vi "r3_Pick&Place_module_chip_Zoffset.vi"() -> ()   [LabVIEW 2016]
uses:
  Classes/Controllers/I-O/Copy of NI-DAQ Folder/NI-DAQ.lvclass
  D:/INTT/V1/Classes/Controllers/I-O/Copy of I-O Folder/I-O.lvclass
  Classes/Controllers/Dispenser/Copy of Ultimus V2 Folder/Ultimus V2.lvclass
  <vilib>/Analysis/coordinate.llb/2D Cartesian Coordinate Rotation (Scalar).vi
  <vilib>/Utility/file.llb/Read Delimited Spreadsheet (DBL).vi
  <vilib>/Utility/file.llb/Write Delimited Spreadsheet (DBL).vi
  Classes/Controllers/Motion/Copy of Motion Folder/Motion.lvclass
  Classes/Controllers/Camera/Copy of Controller Folder/Controller.lvclass
  <vilib>/Analysis/NI_AALPro.lvlib
  Classes/Controllers/I-O/Copy of I-O Folder/I-O.lvclass
panel:
  out "chip place Z offset":dbl[](array[numeric])
  out "air pressure indecator":i32
  in  "glue deposit group":i32=4
  in  "Ultimus Pressure":i16=20
  out "Array 2":dbl[][](array[numeric])
  out "Measured PickupTool position":dbl[][](array[numeric])
  in  "VacChannel for sample":i32=1
  in  "check height? 2":bool
  in  "check height?":bool
  out "Needle parking position":dbl[](array[numeric])
  out "GlueBox":dbl[][](array[numeric])
  out "appended array":dbl[][](array[numeric])
  in  "chip placement height compensation":dbl=-0.47 format="%#_13g"
  out "Sample on HDI":dbl[][](array[numeric]) format="%#_8g"
  in  "Sensor A/B":bool
  out "Gantry current position":dbl[](array[numeric])
  in  "READ Position":bool
  in  "Needle Height Compenstation\n(glue gap)":dbl=0.34
  in  "Needle Alignment":bool
  in  "Parking position":dbl[](array[numeric])=[625.0, 625.0, 0.0, 0.01]
  in  "GOTO":bool
  in  "Default Pickup Tool Position":dbl[][](array[numeric])=[[184.055, 797.167, 41.7168, 0.0130657], [153.043, 779.997, 54.962, 0.0365632]]
  in  "Number of Chips/Sensors \nto be assembled":i32=1
  in  "Default HDI alignment \nmark position":dbl[](array[numeric])=[448.231, 973.808, 78.9737, -3.34415e-05]
  in  "Default HDI size":dbl[](array[numeric])=[24.2991, 231.315, -0.0249987, -3.34415e-05]
  out "# of tasks excuted":i32
  out "Chips on tray position":dbl[][](array[numeric])
  out "measured HDI size":dbl[](array[numeric])
  in  "Chip tray":dbl[](array[numeric])=[465.031, 710.639, 69.8028, 0.00407755]
  out "Sample position \non HDI":dbl[][](array[numeric])
  in  "Inititalize":bool
  in  "Pick and place":bool
  in  "Deposit Glue":bool
  in  "Measure Pickup Tools":bool
  in  "Measure Samples on tray":bool
  out "default chip and sensor position w.r.t. 1st mark":dbl[][](array[numeric])
  in  "Assembly Type":bool=TRUE
  in  "Stop":bool
  in  "Measure HDI":bool
  out "Measure HDI top-left":dbl[](array[numeric])
  # "Chips"
  # "Sensor 0.3 -> 200 micron glue thickness\nChips 0.34-> 150 micron glue thickness"
  # "Sensors"
  # "Sensors B\n(Short)"
  # "Sensors A\n(Long)"
  # "Chips : -0.47-> 60 micron height gap\n               -0.5 -> 90 micron"
  # "ACTIONS"
  # "1"
  # "HDI infomation"
  # "chips use channel 0, 2\nsensors use channel 0, 1"
  # "sensor height 69.8471\nchip height 84.693"
  # "Pick and Place"
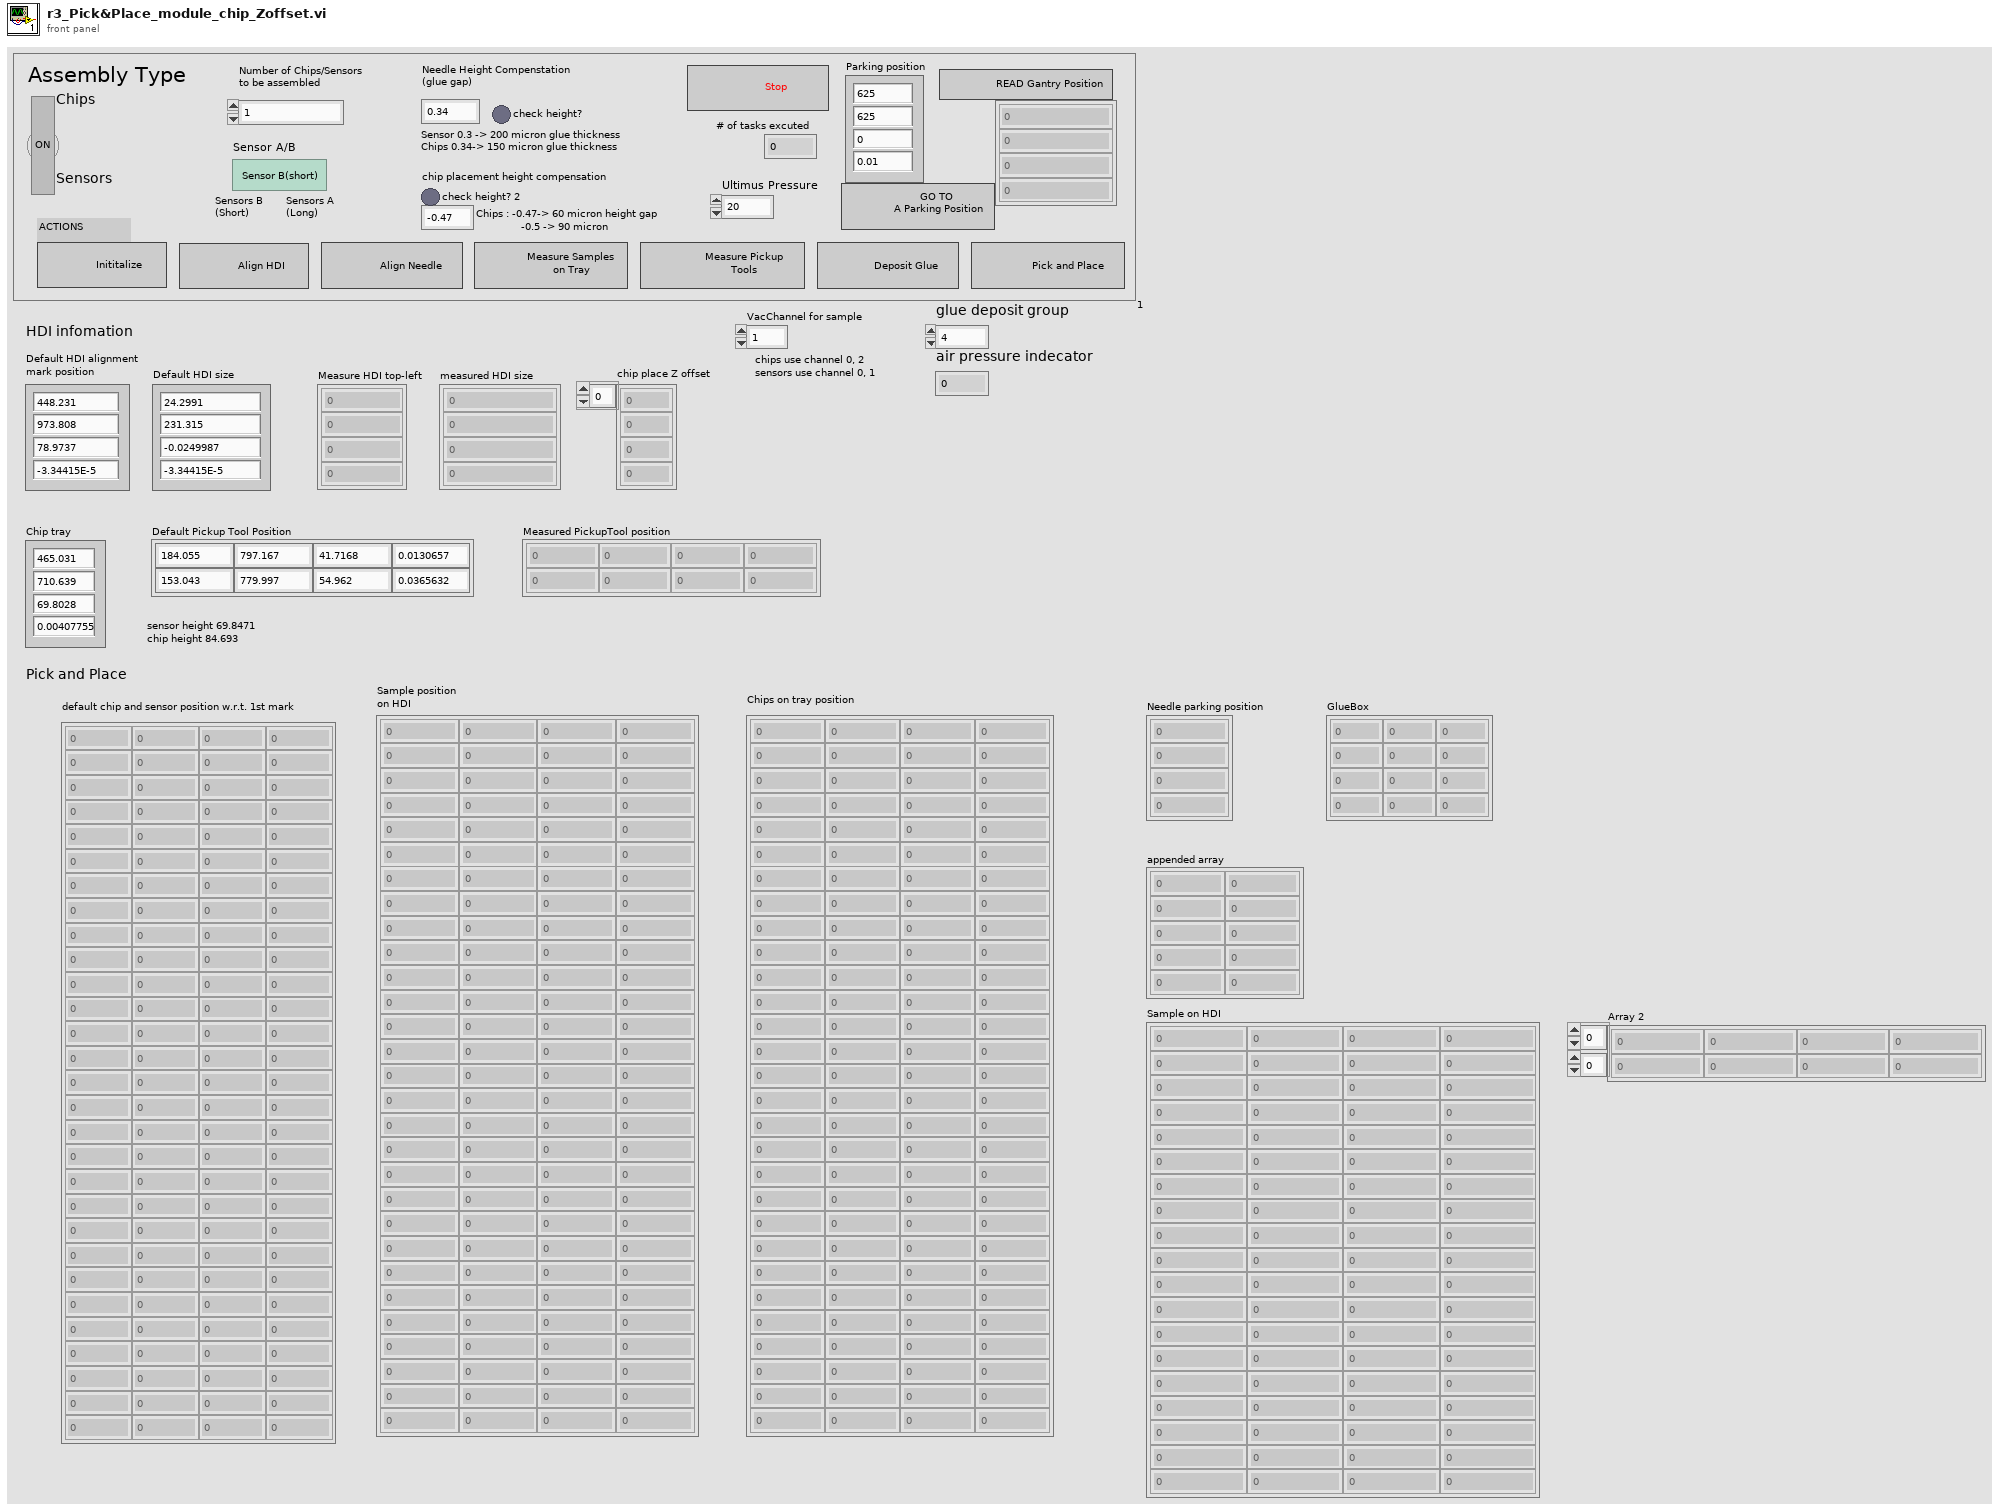
[diagram p1: front panel]
types:
  T1 = typedef "Controller.lvclass/Controllers.ctl" = cluster{"Copy of Motion.lvclass":refnum<class "Motion.lvclass">, "Copy of I-O.lvclass":refnum<class "I-O.lvclass">, "Copy of Dispenser.lvclass":refnum<class "Dispenser.lvclass">}
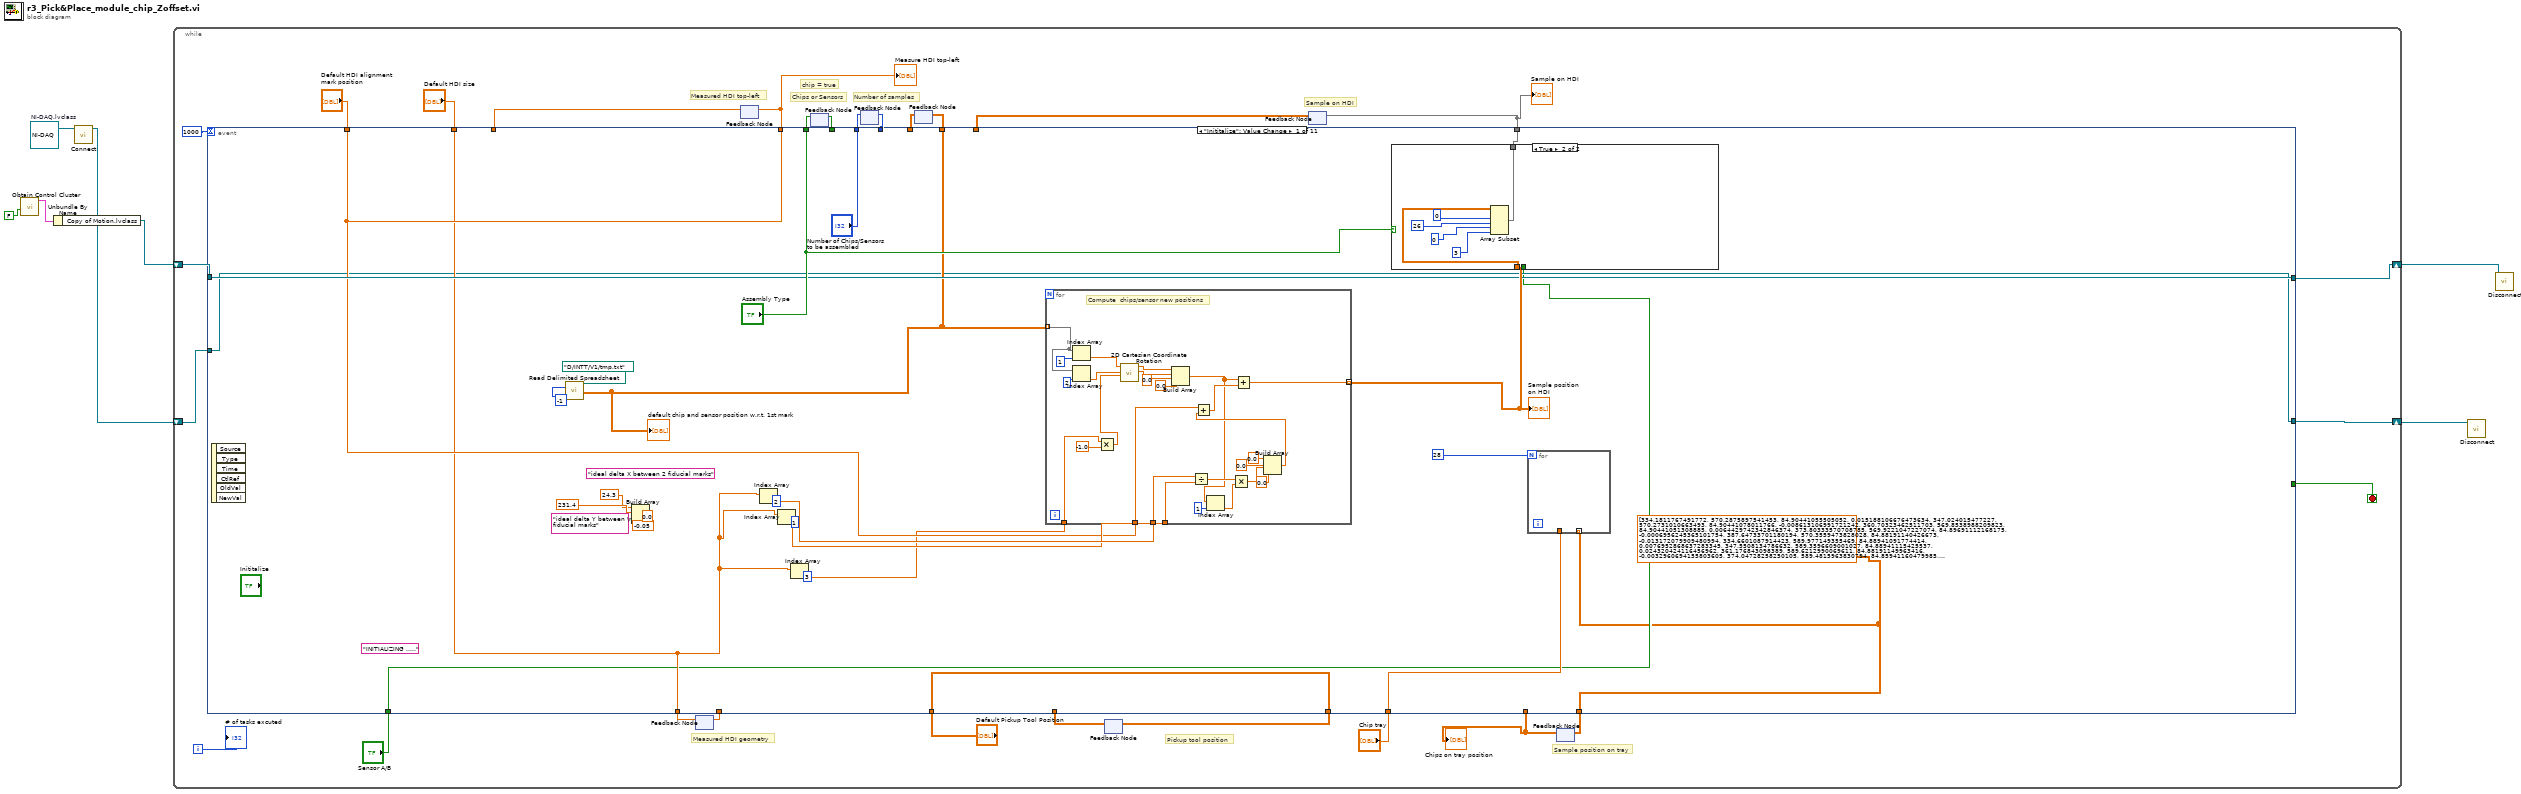
[diagram p0: block diagram]
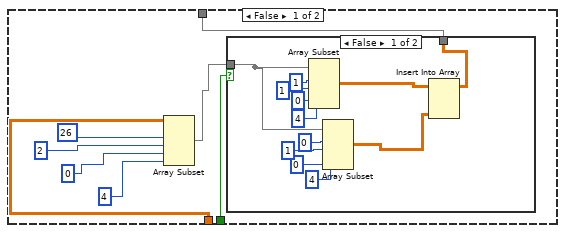
[diagram p2: hidden frame]
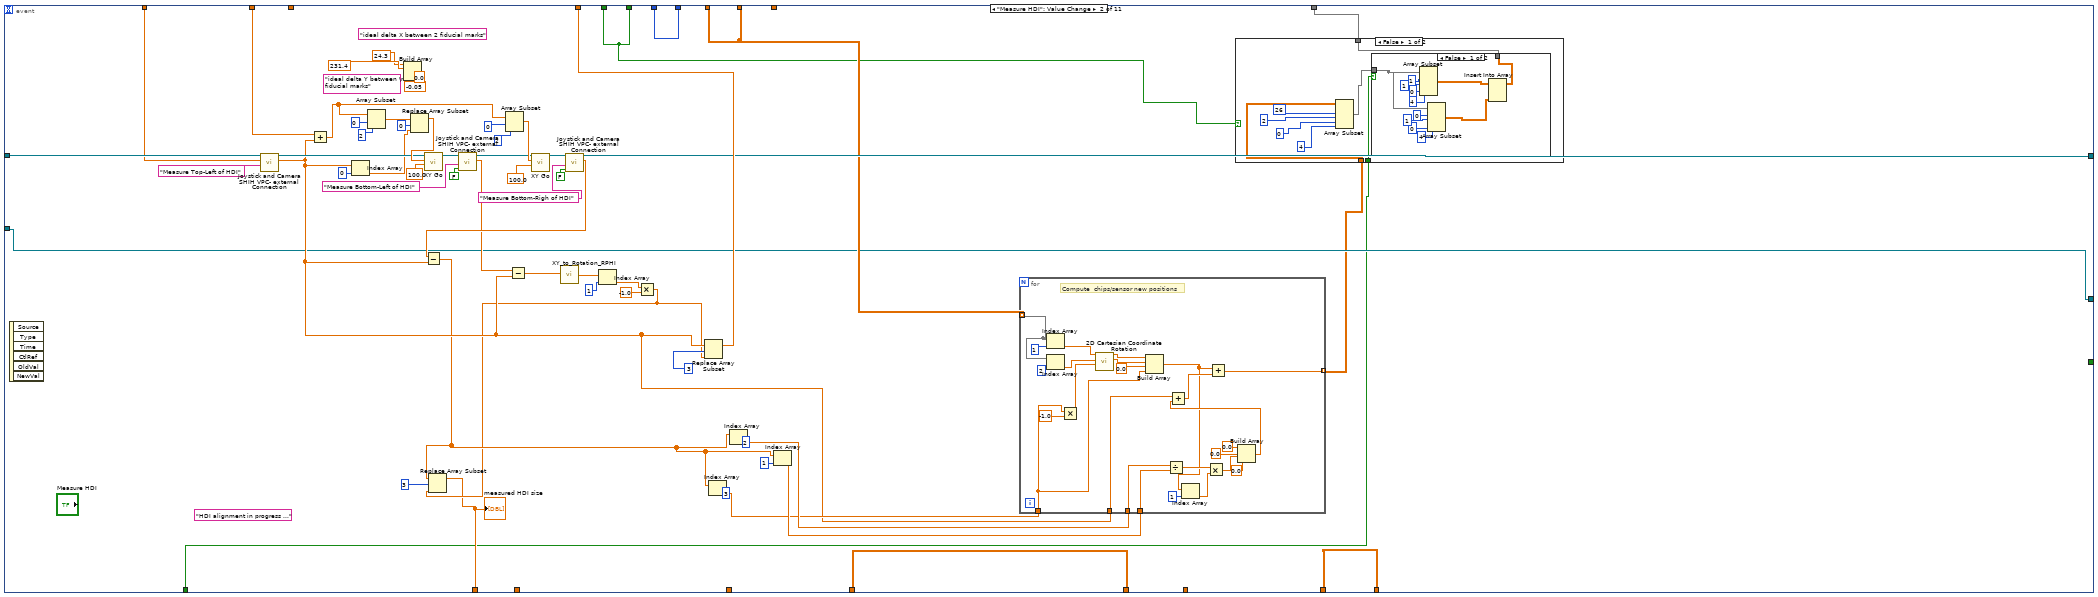
[diagram p4: hidden frame]
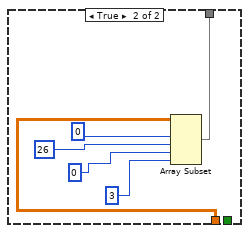
[diagram p6: hidden frame]
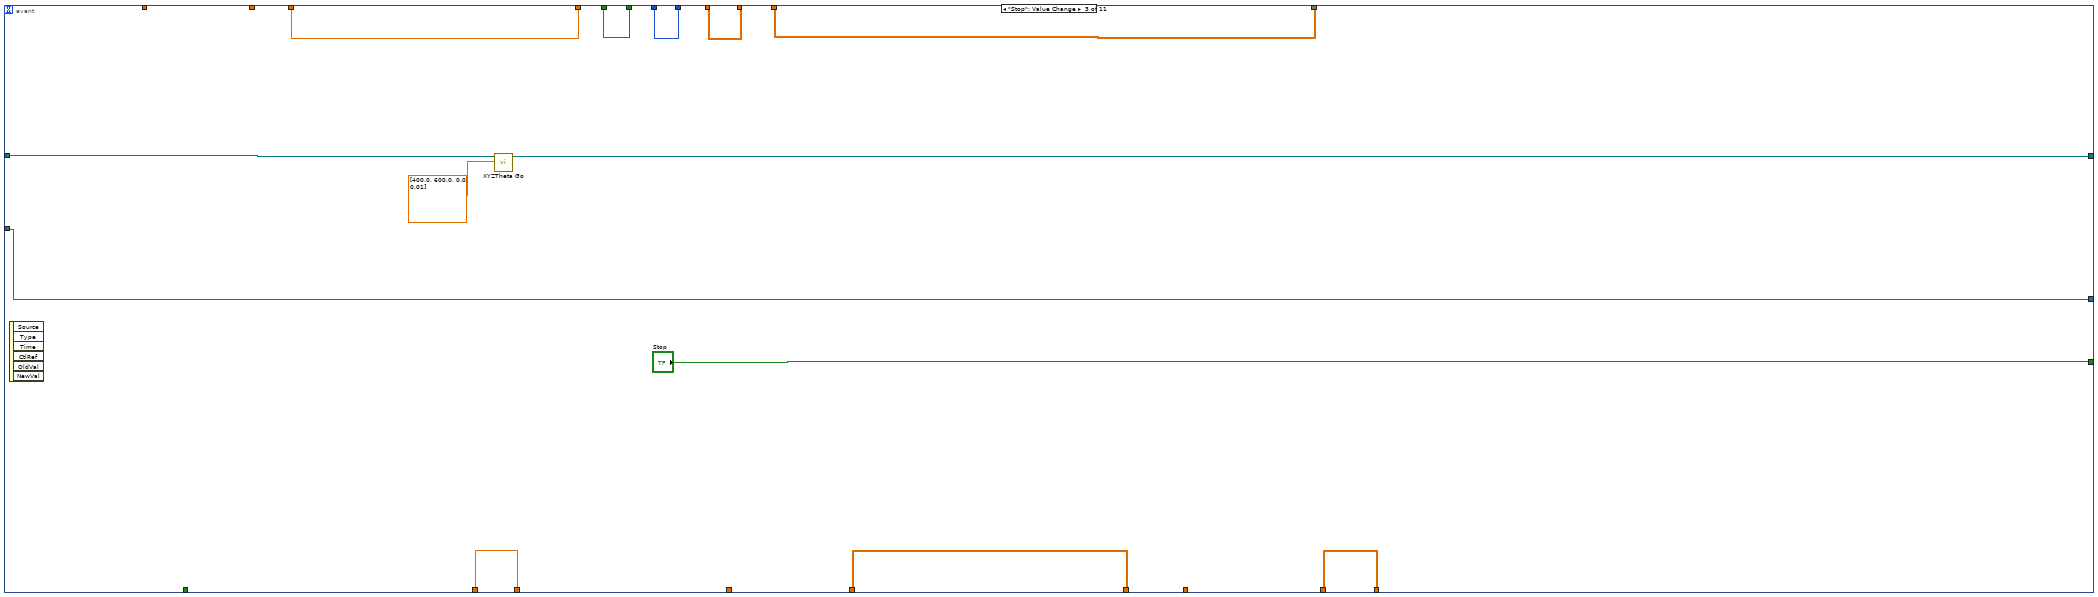
[diagram p7: hidden frame]
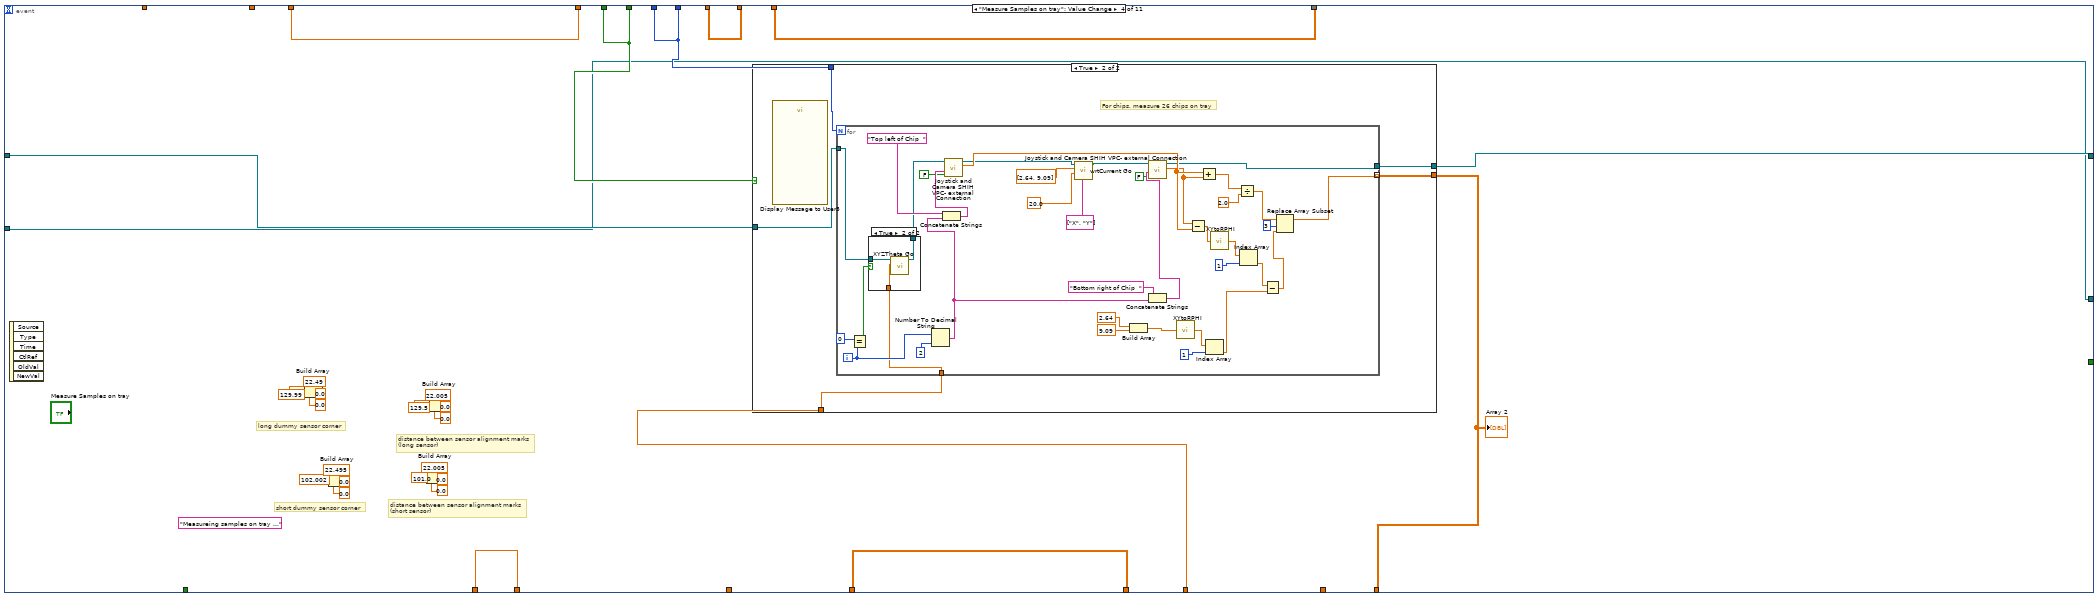
[diagram p8: hidden frame]
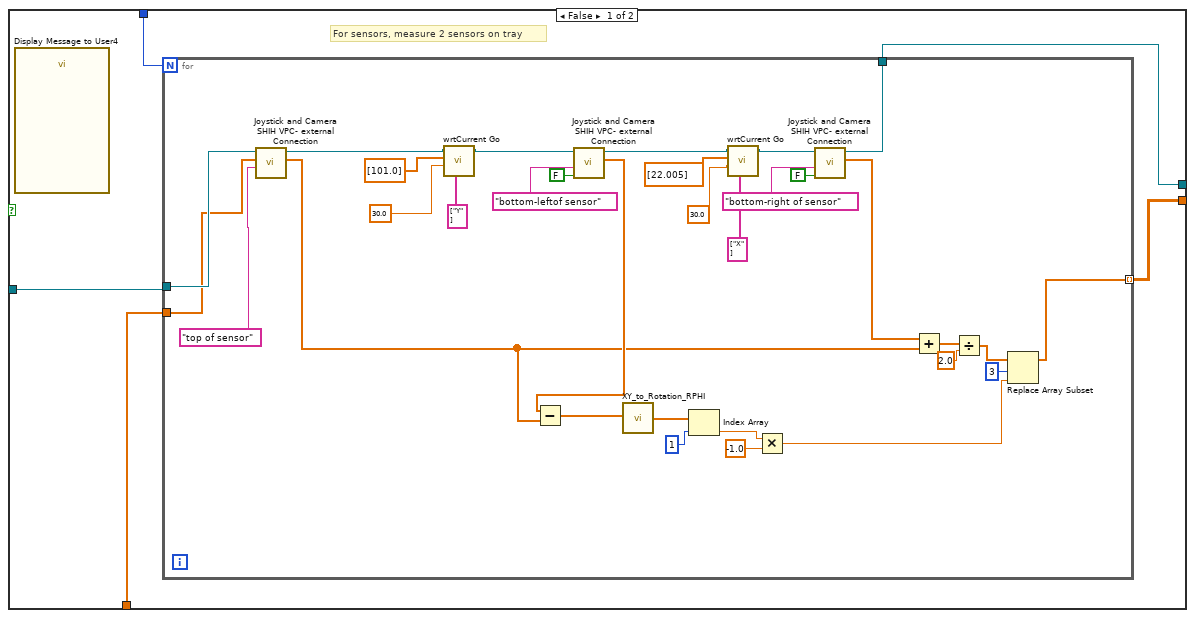
[diagram p9: hidden frame]
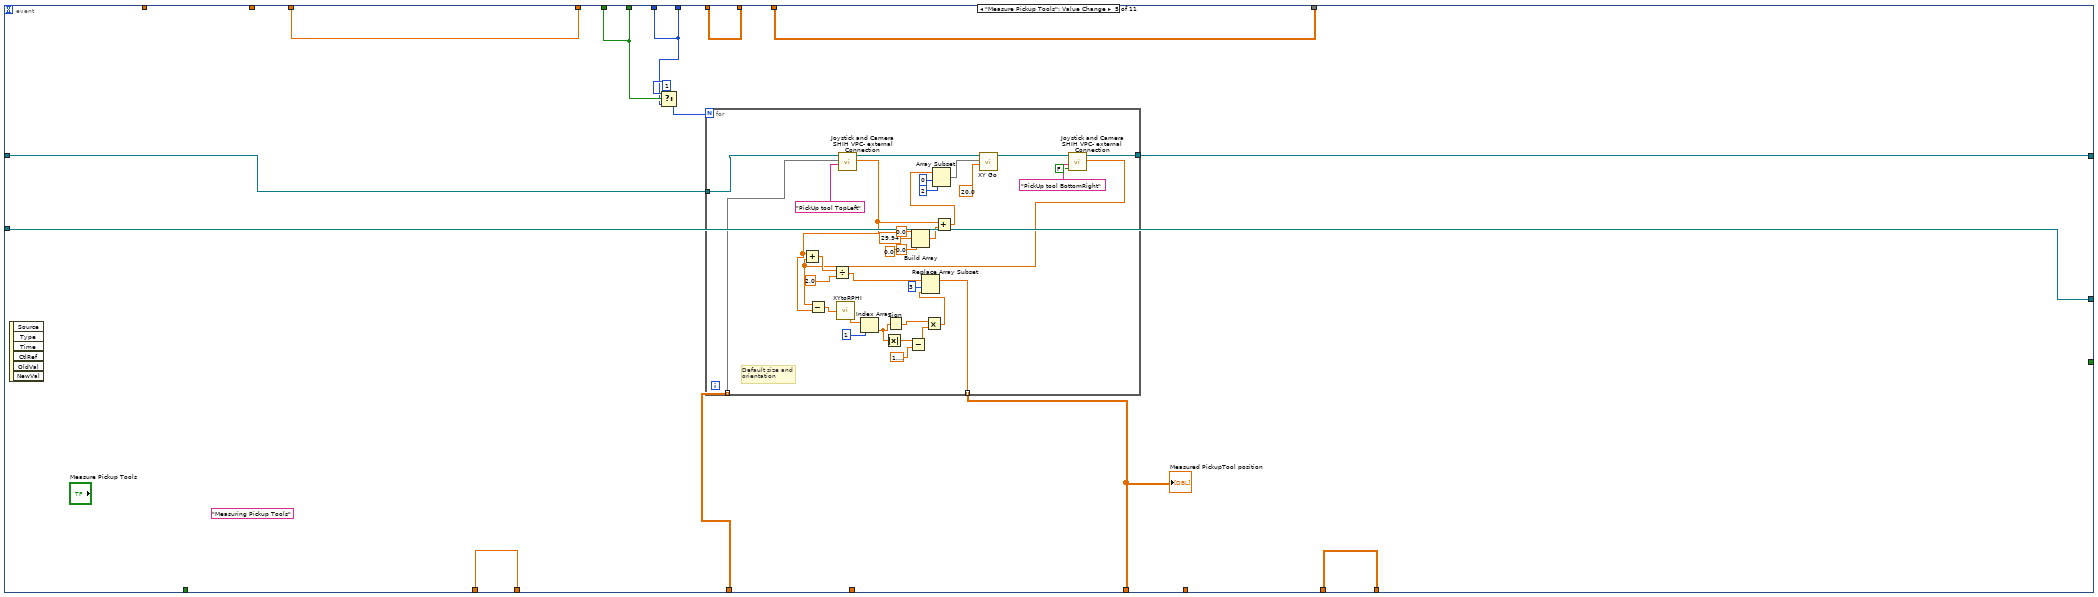
[diagram p11: hidden frame]
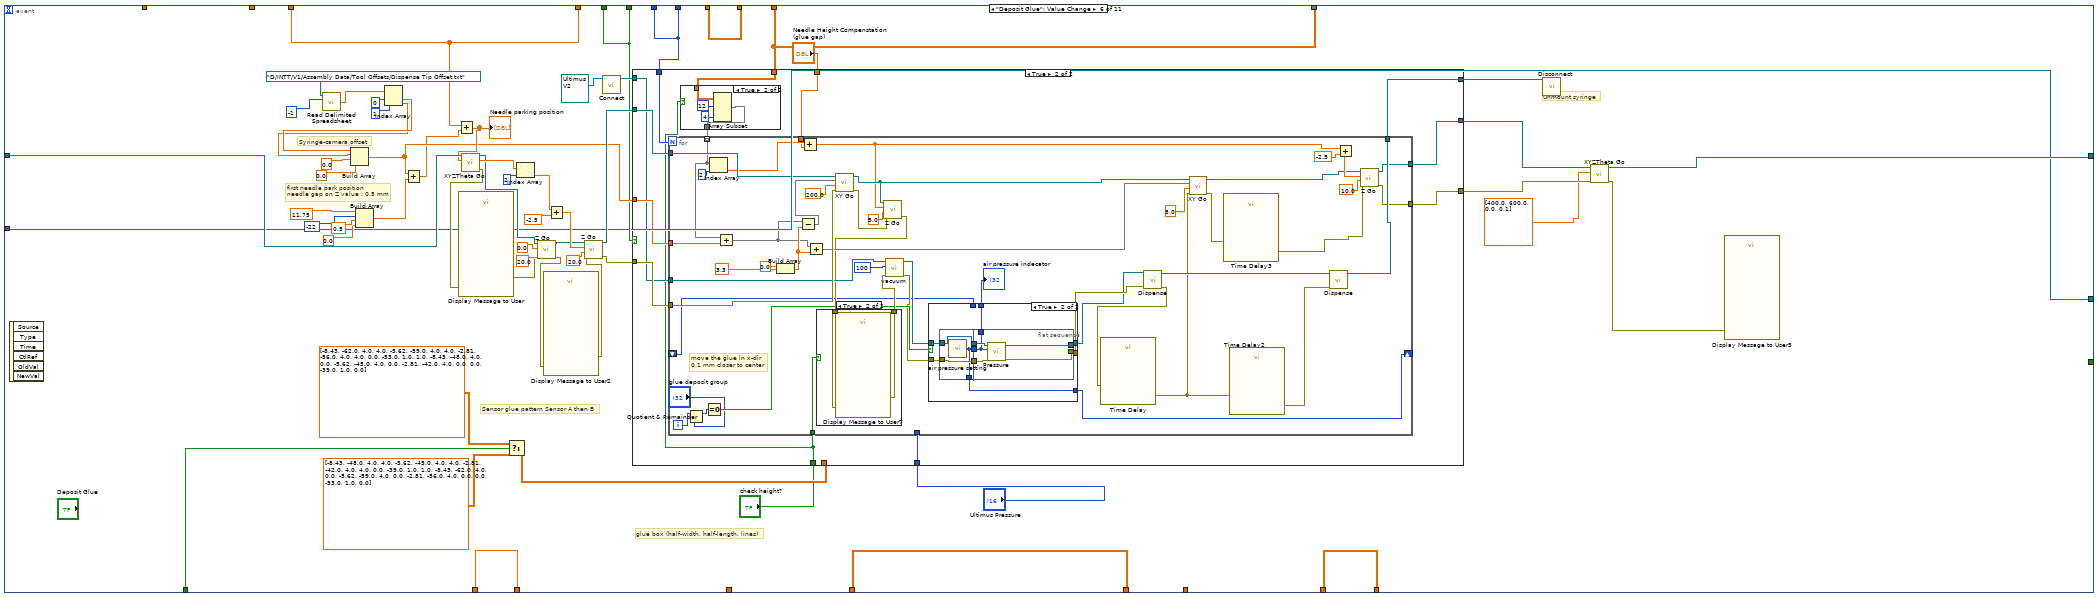
[diagram p12: hidden frame]
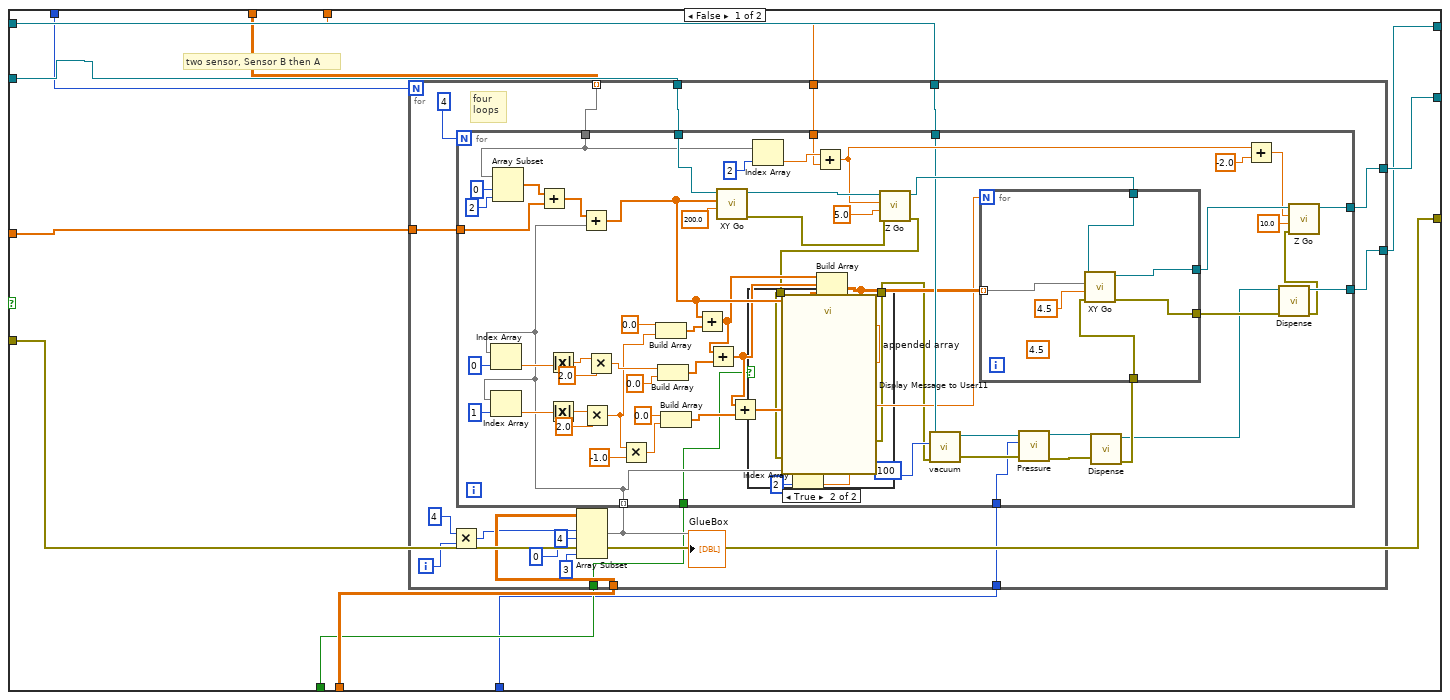
[diagram p13: hidden frame]
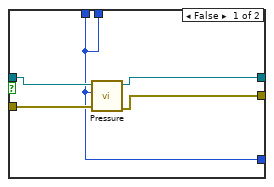
[diagram p16: hidden frame]
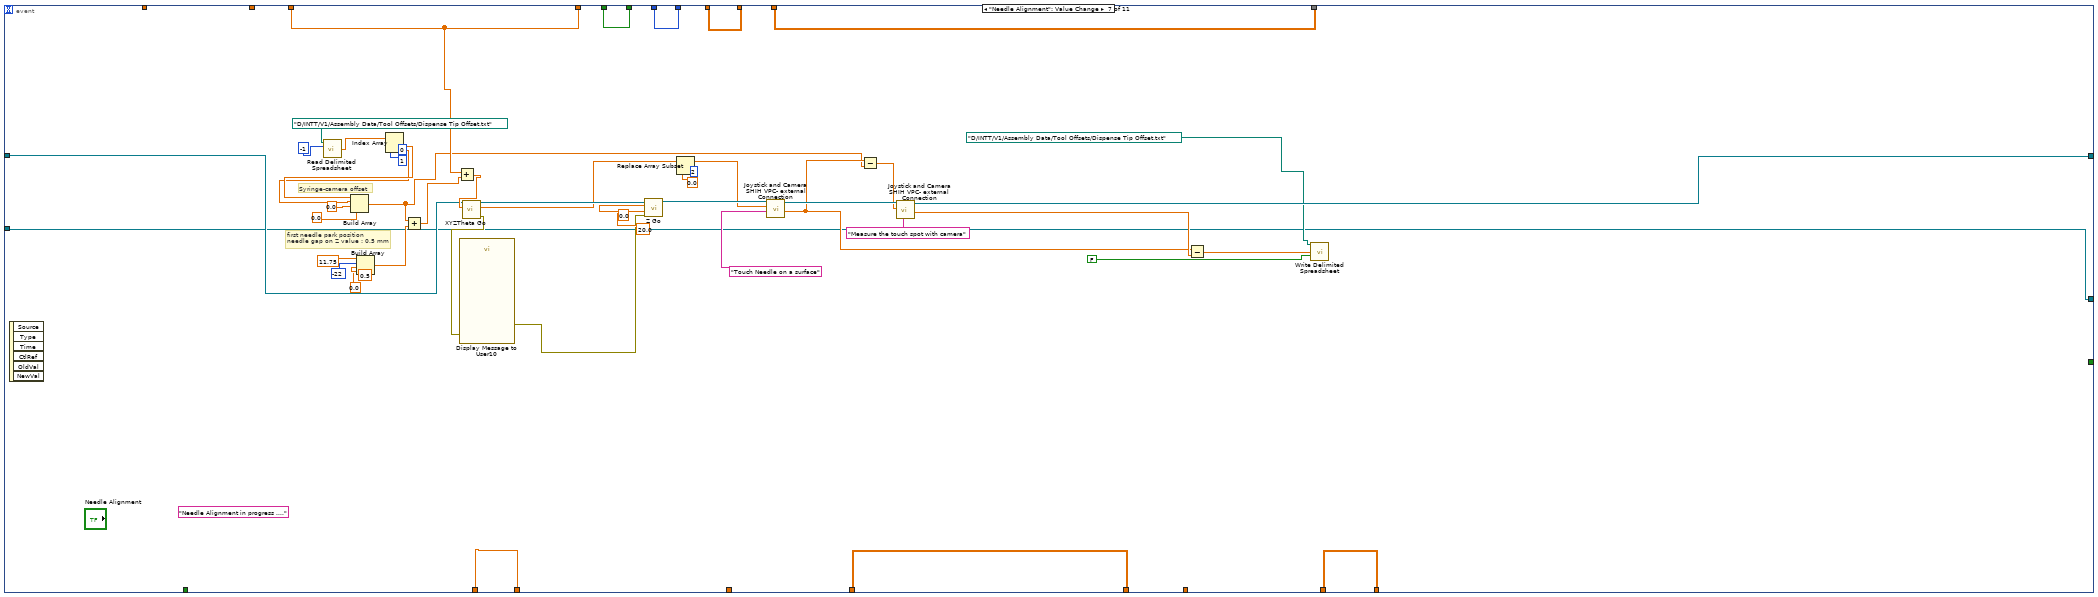
[diagram p18: hidden frame]
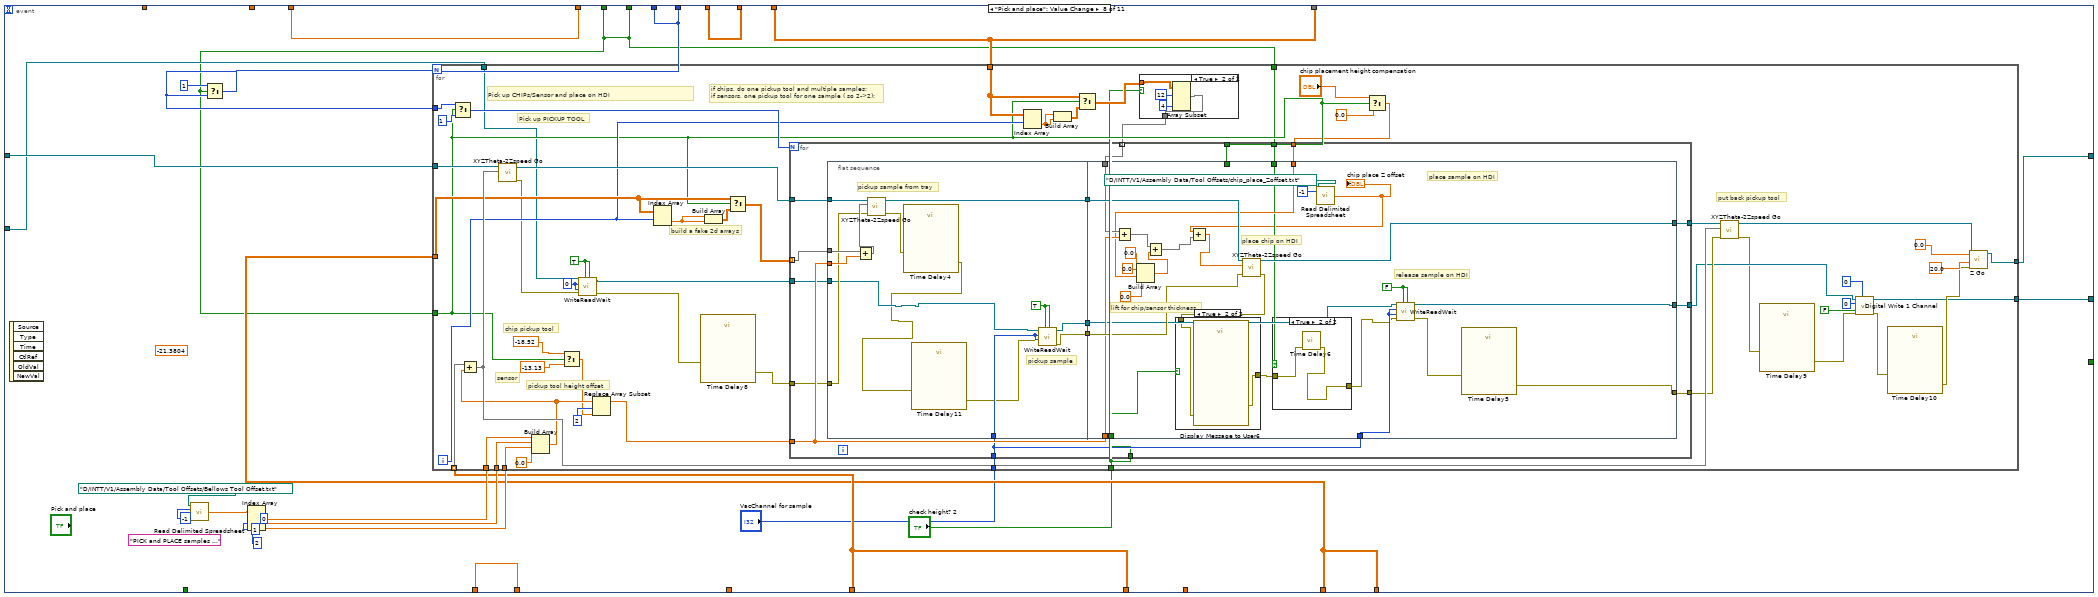
[diagram p19: hidden frame]
diagram:
  w3 = refnum<class "NI-DAQ.lvclass"> refnum  # NI-DAQ.lvclass
  n1 = call "Obtain Control Cluster.vi"("I/O"=FALSE) -> ("Control Out"=w7:T1)  [unwired: 10 in]
  n2 = Unbundle By Name(w7) -> ("Copy of Motion.lvclass"=w5:refnum<class "Motion.lvclass">)
  n3 = call-dynamic "Connect.vi"("NI-DAQ in"=w3) -> ("NI-DAQ out"=w2:refnum<class "NI-DAQ.lvclass">)  [unwired: 9 in, 1 out]
  n4 = while {
    shift-right: [w23] -> w4
    shift-left: w5 -> [w35]
    shift-right: [w9] -> w1
    shift-left: w2 -> [w10]
    i -> [w22]
    stop <- w34 stop-if-true
    # "chip = true"
    # "Pickup tool position"
    # "Chips or Sensors"
    # "Number of samples"
    # "Measured HDI geometry"
    # "Sample position on tray"
    # "Measured HDI top-left"
    # "Sample on HDI"
    n5 = feedback #1() -> (w30:dbl[])  [unwired: 1 in]
    n6 = feedback #2() -> (w32:dbl[])  [unwired: 1 in]
    n7 = feedback #3() -> (w27:bool)  [unwired: 1 in]
    n8 = feedback #4() -> (w21:i32)  [unwired: 1 in]
    n9 = feedback #5() -> (w16:dbl[][])  [unwired: 1 in]
    n10 = feedback #6() -> (w24:dbl[][])  [unwired: 1 in]
    n11 = feedback #7() -> (w29:dbl[][])  [unwired: 1 in]
    n12 = feedback #8() -> (w13:dbl[][])  [unwired: 1 in]
    "Chips on tray position" <- w13
    n13 = event shown="[0] \"Inititalize\": Value Change" {
      selector: _ -> [_ _ _ _ _ _ _ _ _ _ _]
      dyn-events: _ -> [_ _ _ _ _ _ _ _ _ _ _]
      timeout: 1000 -> [_ _ _ _ _ _ _ _ _ _ _]
      tunnel: w35 -> [w48 w173 w238 w266 w363 w431 w666 w718 w849 w870 w872]
      tunnel: [_ _ "Stop" _ _ _ _ _ _ _ _] -> w34
      tunnel: [w45 w170 w231 w260 w354 w412 w674 w702 w858 w864 w880] -> w33
      tunnel: w32 -> [_ _ w231 w260 w354 w412 w674 w702 w858 w864 w880]
      tunnel: ["Assembly Type" w117 w235 w264 w359 w415 w673 w696 w857 w865 w879] -> w28
      tunnel: [w41 w120 w230 w259 w353 w408 w669 w701 w853 w863 w873] -> w31
      tunnel: w30 -> [_ _ w230 w259 w353 w408 w669 w701 w853 w863 w873]
      tunnel: [w37 w118 w232 w261 w356 w414 w670 w707 w854 w868 w876] -> w11
      tunnel: w29 -> [_ _ w232 w261 w356 w414 w670 w707 w854 w868 w876]
      tunnel: w27 -> [_ w117 w235 w264 w359 w415 w673 w696 w857 w865 w879]
      tunnel: w21 -> [_ w161 w234 w263 w358 w413 w672 w704 w856 w866 w878]
      tunnel: [w36 w159 w228 w240 w352 w410 w667 w705 w851 w861 w875] -> w26
      tunnel: w13 -> [_ w159 w228 _ w352 w410 w667 w705 w851 w861 w875]
      tunnel: [w44 w160 w229 w258 w362 w409 w668 w706 w852 w862 w874] -> w25
      tunnel: w24 -> [_ w160 w229 w258 _ w409 w668 w706 w852 w862 w874]
      tunnel: [w48 w169 w236 w265 w361 w416 w658 w708 w848 w869 w872] -> w23
      tunnel: ["Number of Chips/Sensors \nto be assembled" w161 w234 w263 w358 w413 w672 w704 w856 w866 w878] -> w20
      tunnel: "Default HDI alignment \nmark position" -> [w45 w168 _ _ _ _ _ _ _ _ _]
      tunnel: "Default HDI size" -> [w41 w167 _ _ _ _ _ _ _ _ _]
      tunnel: [w46 w162 w233 w262 w355 w407 w671 w703 w855 w867 w877] -> w17
      tunnel: w16 -> [_ w162 w233 w262 w355 w407 w671 w703 w855 w867 w877]
      tunnel: "Default Pickup Tool Position" -> [w44 _ _ _ w357 _ _ _ _ _ _]
      tunnel: "Chip tray" -> [w43 _ _ w257 _ _ _ _ _ _ _]
      tunnel: "Sensor A/B" -> [w38 w115 _ _ _ w406 _ _ _ _ _]
      tunnel: w10 -> [w39 w119 w226 w239 w351 w400 w649 w699 w850 w859 w871]
      tunnel: [w39 w119 w226 w239 w351 w400 w649 w700 w850 w859 w871] -> w9
      event "Inititalize": Value Change {
        w36 = dbl[][] [[334.1811767491772, 570.2875897541453, 84.90441055505052, 0.015188106676473634], [347.024015477227, 570.2731010663493, 84.90441078011766, -0.008613106991721242], [360.70323462511703, 569.8538988209823, 84.90441051308885, 0.0064429742342846374], [373.80333570708785, 569.9221047227074, 84.89691112168175, -0.0006956245365101754], [387.64733701180194, 570.3559473828028, 84.88191140426673, -0.013172079909480994], [334.6601087914423, 589.977149355469, 84.88941091774414, 0.0076952868637283345], [347.5508134786632, 589.3596609001027, 84.88941115425537, 0.024320424116456962], [361.176843098389, 589.6212990069611, 84.88191149963416, -0.0032960694155803605], [374.04728258250105, 589.4815963830794, 84.85941160479985, 0.010838192817480552], [387.4497250921253, 589.6538201535805, 84.82941149439927, -0.03343715590492602], [333.55852334776785, 609.5455685376184, 84.90440689146459, -0.018311916571119413], [347.7966033216097, 608.6437844720085, 84.87440757870488, -0.015752079606068392], [361.4949227393362, 608.7813796953453, 84.85940765129695, -0.01604506442231468], [333.7785290001573, 629.3200126889597, 84.87440547988311, 0.005904682283682794], [347.51213526180516, 629.7480723097874, 84.87440578505888, -0.009605828526077165], [361.27882752559685, 629.3502048357473, 84.85940509834163, -0.0041409175627777906], [374.7088143795405, 629.2749076489376, 84.84440562125255, -0.014408155589034077], [387.20468481334456, 629.6557649943925, 84.81440540404043, -0.00563941201623841], [335.45377050885696, 649.7886349362416, 84.90439972487917, -0.009188371633077175], [347.4946640880062, 650.0246528581602, 84.90439958373537, -0.00842603609961845], [361.67790069553246, 650.2275573255758, 84.88189946364935, -0.016787416223704943], [375.5468303171785, 649.8722061399783, 84.8668997271829, 0.018058031233532557], [387.4479197331095, 650.625158025664, 84.85940009924254, -0.004760316868086312], [334.4843305025747, 669.0027249305689, 84.91939588588893, -0.0007289518392163963], [347.7040517829141, 668.7207175623021, 84.91939637035549, 0.009671429582633673], [361.3137955038096, 668.6488204230046, 84.9193962139529, 0.009801952697993555]] ("Chips on tray position")
        (unwired) "INITIALIZING ....." ("String")
        (unwired) "ideal delta Y between \n2 fiducial marks"
        (unwired) "ideal delta X between 2 fiducial marks"
        n14 = event-data() -> ()  [unwired: 1 in, 6 out]
        n15 = call-poly <vilib>:"Read Delimited Spreadsheet.vi"("file path (dialog if empty)"=path "D:/INTT/V1/tmp.txt", "number of rows (all:-1)"=-1) -> ("all rows"=w46:dbl[][])  [unwired: 8 in, 5 out]
        "default chip and sensor position w.r.t. 1st mark" <- w46
        n16 = Build Array(24.3 ("y"), 231.4 ("y"), 0.0 ("element"), -0.05 ("element")) -> ()  [unwired: 1 out]
        n17 = Index Array(array=w41, index=2) -> (element=w57:dbl)
        n18 = Index Array(array=w41, index=1) -> (element=w56:dbl)
        n19 = Index Array(array=w41, index=3) -> (element=w40:dbl)
        n20 = for {
          tunnel: w46 -> [w107] mode=indexing
          tunnel: w40 -> [w90]
          tunnel: w45 -> [w99]
          tunnel: [w106] -> w50 mode=indexing
          tunnel: w57 -> [w105]
          tunnel: w56 -> [w96]
          # "Compute  chips/sensor new positions"
          n21 = Index Array(array=w107, index=1) -> (element=w111:dbl)
          n22 = Index Array(array=w107, index=2) -> (element=w110:dbl)
          n23 = Multiply(x=w90, y=-1.0) -> (x*y=w91:dbl)
          n24 = call-poly <vilib>:"2D Cartesian Coordinate Rotation.vi"("theta"=w91, "y"=w110, "x"=w111) -> ("y out"=w113:dbl, "x out"=w112:dbl)  [unwired: 6 in, 1 out]
          n25 = Build Array(w112, w113, 0.0 ("element"), 0.0 ("element")) -> (w93:dbl[])
          n26 = Divide(x=w105, y=w96) -> (x/y=w104:dbl)
          n27 = Index Array(array=w93, index=1) -> (element=w94:dbl)
          n28 = Multiply(x=w104, y=w94) -> (x*y=w100:dbl)
          n29 = Build Array(0.0 ("element"), 0.0 ("element"), w100, 0.0 ("element")) -> (w98:dbl[])
          n30 = Add(x=w99, y=w98) -> (x+y=w97:dbl[])
          n31 = Add(x=w93, y=w97) -> (x+y=w106:dbl[])
        }
        "Sample position \non HDI" <- w50
        n32 = case shown="True" "Assembly Type" {
          tunnel: w50 -> [w65 w85]
          tunnel: [w63 w83] -> w37
          tunnel: w38 -> [w62 _]
          frame False {
            n33 = Array Subset(array=w65, index (row)=26 ("index"), length (row)=2 ("length"), index (col)=0, length (col)=4 ("length")) -> (w64:dbl[][])
            n34 = case shown="False" w62 {
              tunnel: w64 -> [w73 w82]
              tunnel: [w70 w82] -> w63
              frame False {
                n35 = Array Subset(array=w73, index (row)=1 ("index"), length (row)=1 ("length"), index (col)=0 ("index"), length (col)=4 ("length")) -> (w72:dbl[][])
                n36 = Array Subset(array=w73, index (row)=0 ("index"), length (row)=1 ("length"), index (col)=0 ("index"), length (col)=4 ("length")) -> (w71:dbl[][])
                n37 = Insert Into Array(array=w72, new element=w71) -> (w70:dbl[][])  [unwired: 2 in]
              }
              frame True {
              }
            }
          }
          frame True {
            n38 = Array Subset(array=w85, index (row)=0 ("index"), length (row)=26 ("length"), index (col)=0, length (col)=3 ("length")) -> (w83:dbl[][])
          }
        }
        n39 = for {
          N: 28 -> [_]
          tunnel: w43 -> [_]
          tunnel: w36 -> [_] mode=indexing
        }
      }
      event "Measure HDI": Value Change {
        (unwired) "ideal delta Y between \n2 fiducial marks"
        (unwired) "ideal delta X between 2 fiducial marks"
        (unwired) "HDI alignment in progress ..." ("String")
        n40 = event-data() -> ()  [unwired: 1 in, 6 out]
        n41 = call "Joystick and Camera SHIH VPC- external Connection.vi"("Motion in"=w173, "XYZTheta"=w168, "Measurement Point"="Measure Top-Left of HDI") -> ("Motion out"=w137:refnum<class "Motion.lvclass">, "Sum"=w126:dbl[])  [unwired: 4 in, 2 out]
        n42 = Add(x=w167, y=w126) -> (x+y=w141:dbl[])
        n43 = Index Array(array=w126, index=0) -> (element=w128:dbl)
        n44 = Array Subset(array=w141, index=0, length=2) -> (w140:dbl[])
        n45 = Build Array(24.3 ("y"), 231.4 ("y"), 0.0 ("element"), -0.05 ("element")) -> ()  [unwired: 1 out]
        n46 = Replace Array Subset(array=w140, new element=w128, index=0) -> (w138:dbl[])
        n47 = call-dynamic "XY Go.vi"("Speed"=100.0, "XY"=w138, "Motion in"=w137) -> ("Motion out"=w145:refnum<class "Motion.lvclass">)  [unwired: 7 in, 1 out]
        n48 = call "Joystick and Camera SHIH VPC- external Connection.vi"("Motion in"=w145, "Measurement Point"="Measure Bottom-Left of HDI", "Inital GO"=FALSE) -> ("Motion out"=w136:refnum<class "Motion.lvclass">, "Sum"=w127:dbl[])  [unwired: 4 in, 2 out]
        n49 = Array Subset(array=w141, index=0, length=2) -> (w151:dbl[])
        n50 = Subtract(x=w127, y=w126) -> (x-y=w135:dbl[])
        n51 = call-dynamic "XY Go.vi"("Speed"=100.0, "XY"=w151, "Motion in"=w136) -> ("Motion out"=w155:refnum<class "Motion.lvclass">)  [unwired: 7 in, 1 out]
        n52 = call "XY_to_Rotation_RPHI.vi"("X-Y"=w135) -> ("r-phi"=w131:dbl[])
        n53 = call "Joystick and Camera SHIH VPC- external Connection.vi"("Motion in"=w155, "Measurement Point"="Measure Bottom-Righ of HDI", "Inital GO"=FALSE) -> ("Motion out"=w169:refnum<class "Motion.lvclass">, "Sum"=w172:dbl[])  [unwired: 4 in, 2 out]
        n54 = Subtract(x=w172, y=w126) -> (x-y=w123:dbl[])
        n55 = Index Array(array=w131, index=1) -> (element=w124:dbl)
        n56 = Multiply(x=w124, y=-1.0) -> (x*y=w121:dbl)
        n57 = Replace Array Subset(array=w123, new element=w121, index=3) -> (w120:dbl[])
        "measured HDI size" <- w120
        n58 = Replace Array Subset(array=w126, new element=w121, index=3) -> (w170:dbl[])
        n59 = Index Array(array=w123, index=3) -> (element=w157:dbl)
        n60 = Index Array(array=w123, index=2) -> (element=w164:dbl)
        n61 = Index Array(array=w123, index=1) -> (element=w163:dbl)
        n62 = for {
          tunnel: w162 -> [w218] mode=indexing
          tunnel: w157 -> [w202]
          tunnel: w126 -> [w210]
          tunnel: [w217] -> w116 mode=indexing
          tunnel: w164 -> [w216]
          tunnel: w163 -> [w207]
          # "Compute  chips/sensor new positions"
          n63 = Index Array(array=w218, index=1) -> (element=w222:dbl)
          n64 = Index Array(array=w218, index=2) -> (element=w221:dbl)
          n65 = Multiply(x=w202, y=-1.0) -> (x*y=w201:dbl)
          n66 = call-poly <vilib>:"2D Cartesian Coordinate Rotation.vi"("theta"=w201, "y"=w221, "x"=w222) -> ("y out"=w224:dbl, "x out"=w223:dbl)  [unwired: 6 in, 1 out]
          n67 = Build Array(w223, w224, 0.0 ("element"), w202) -> (w204:dbl[])
          n68 = Divide(x=w216, y=w207) -> (x/y=w215:dbl)
          n69 = Index Array(array=w204, index=1) -> (element=w205:dbl)
          n70 = Multiply(x=w215, y=w205) -> (x*y=w211:dbl)
          n71 = Build Array(0.0 ("element"), 0.0 ("element"), w211, 0.0 ("element")) -> (w209:dbl[])
          n72 = Add(x=w210, y=w209) -> (x+y=w208:dbl[])
          n73 = Add(x=w204, y=w208) -> (x+y=w217:dbl[])
        }
        n74 = case shown="False" w117 {
          tunnel: w116 -> [w177 w197]
          tunnel: [w175 w195] -> w118
          tunnel: w115 -> [w174 _]
          frame False {
            n75 = Array Subset(array=w177, index (row)=26 ("index"), length (row)=2 ("length"), index (col)=0, length (col)=4 ("length")) -> (w176:dbl[][])
            n76 = case shown="False" w174 {
              tunnel: w176 -> [w185 w194]
              tunnel: [w182 w194] -> w175
              frame False {
                n77 = Array Subset(array=w185, index (row)=1 ("index"), length (row)=1 ("length"), index (col)=0 ("index"), length (col)=4 ("length")) -> (w184:dbl[][])
                n78 = Array Subset(array=w185, index (row)=0 ("index"), length (row)=1 ("length"), index (col)=0 ("index"), length (col)=4 ("length")) -> (w183:dbl[][])
                n79 = Insert Into Array(array=w184, new element=w183) -> (w182:dbl[][])  [unwired: 2 in]
              }
              frame True {
              }
            }
          }
          frame True {
            n80 = Array Subset(array=w197, index (row)=0 ("index"), length (row)=26 ("length"), index (col)=0, length (col)=3 ("length")) -> (w195:dbl[][])
          }
        }
      }
      event "Stop": Value Change {
        n81 = event-data() -> ()  [unwired: 1 in, 6 out]
        n82 = call "XYZTheta Go.vi"("XYZTheta In"=dbl[] [400.0, 600.0, 0.0, 0.01], "Motion in"=w238) -> ("Motion out"=w236:refnum<class "Motion.lvclass">)  [unwired: 7 in, 2 out]
      }
      event "Measure Samples on tray": Value Change {
        (unwired) "Measureing samples on tray ..." ("String")
        # "long dummy sensor corner"
        # "short dummy sensor corner"
        # "distance between sensor alignment marks\n(short sensor)"
        # "distance between sensor alignment marks\n(long sensor)"
        n83 = event-data() -> ()  [unwired: 1 in, 6 out]
        n84 = Build Array(22.49 ("element"), 129.99 ("element"), 0.0 ("element"), 0.0 ("element")) -> ()  [unwired: 1 out]
        n85 = Build Array(22.495 ("element"), 102.002 ("element"), 0.0 ("element"), 0.0 ("element")) -> ()  [unwired: 1 out]
        n86 = Build Array(22.005 ("element"), 101.0 ("element"), 0.0 ("element"), 0.0 ("element")) -> ()  [unwired: 1 out]
        n87 = Build Array(22.005 ("element"), 129.5 ("element"), 0.0 ("element"), 0.0 ("element")) -> ()  [unwired: 1 out]
        n88 = case shown="True" w264 {
          tunnel: [w268 w308] -> w240
          tunnel: w266 -> [w271 w307]
          tunnel: [w267 w306] -> w265
          tunnel: w263 -> [w270 w305]
          tunnel: w257 -> [w269 w304]
          frame False {
            # "For sensors, measure 2 sensors on tray"
            n89 = call "Display Message to User4"() -> ()  [unwired: 10 in, 2 out]
            n90 = for {
              N: w270 -> [_]
              tunnel: w271 -> [w303]
              tunnel: [w300] -> w267
              tunnel: [w294] -> w268 mode=indexing
              tunnel: w269 -> [w293]
              n91 = call "Joystick and Camera SHIH VPC- external Connection.vi"("Motion in"=w303, "XYZTheta"=w293, "Measurement Point"="top of sensor") -> ("Motion out"=w275:refnum<class "Motion.lvclass">, "Sum"=w282:dbl[])  [unwired: 4 in, 2 out]
              n92 = call-dynamic "wrtCurrent Go.vi"("axis names"=string[] ["Y"], "Speed"=30.0, "distances"=dbl[] [101.0], "Motion in"=w275) -> ("Motion out"=w274:refnum<class "Motion.lvclass">)  [unwired: 6 in, 1 out]
              n93 = call "Joystick and Camera SHIH VPC- external Connection.vi"("Motion in"=w274, "Measurement Point"="bottom-leftof sensor", "Inital GO"=FALSE) -> ("Motion out"=w280:refnum<class "Motion.lvclass">, "Sum"=w284:dbl[])  [unwired: 4 in, 2 out]
              n94 = Subtract(x=w284, y=w282) -> (x-y=w289:dbl[])
              n95 = call "XY_to_Rotation_RPHI.vi"("X-Y"=w289) -> ("r-phi"=w288:dbl[])
              n96 = Index Array(array=w288, index=1) -> (element=w285:dbl)
              n97 = call-dynamic "wrtCurrent Go.vi"("axis names"=string[] ["X"], "Speed"=30.0, "distances"=dbl[] [22.005], "Motion in"=w280) -> ("Motion out"=w281:refnum<class "Motion.lvclass">)  [unwired: 6 in, 1 out]
              n98 = Multiply(x=w285, y=-1.0) -> (x*y=w283:dbl)
              n99 = call "Joystick and Camera SHIH VPC- external Connection.vi"("Motion in"=w281, "Measurement Point"="bottom-right of sensor", "Inital GO"=FALSE) -> ("Motion out"=w300:refnum<class "Motion.lvclass">, "Sum"=w297:dbl[])  [unwired: 4 in, 2 out]
              n100 = Add(x=w297, y=w282) -> (x+y=w298:dbl[])
              n101 = Divide(x=w298, y=2.0) -> (x/y=w296:dbl[])
              n102 = Replace Array Subset(array=w296, new element=w283, index=3) -> (w294:dbl[])
            }
          }
          frame True {
            # "For chips, measure 26 chips on tray"
            n103 = call "Display Message to User5"() -> ()  [unwired: 10 in, 2 out]
            n104 = for {
              N: w305 -> [_]
              tunnel: [w335] -> w308 mode=indexing
              tunnel: w307 -> [w319]
              tunnel: [w315] -> w306
              tunnel: w304 -> [w320]
              i -> [w323]
              n105 = Equal?(x=0, y=w323) -> (x = y?=w321:bool)
              n106 = case shown="True" w321 {
                tunnel: w320 -> [_ w350]
                tunnel: w319 -> [w347 w349]
                tunnel: [w347 w348] -> w318
                frame False {
                }
                frame True {
                  n107 = call "XYZTheta Go.vi"("XYZTheta In"=w350, "Motion in"=w349) -> ("Motion out"=w348:refnum<class "Motion.lvclass">)  [unwired: 7 in, 2 out]
                }
              }
              n108 = Number To Decimal String(number=w323, width (-)=i16 2) -> (decimal integer string=w339:string)
              n109 = Concatenate Strings("Top left of Chip  " ("string"), w339) -> (w333:string)
              n110 = call "Joystick and Camera SHIH VPC- external Connection.vi"("Motion in"=w318, "Measurement Point"=w333, "Inital GO"=FALSE) -> ("Motion out"=w312:refnum<class "Motion.lvclass">, "Sum"=w338:dbl[])  [unwired: 4 in, 2 out]
              n111 = call-dynamic "wrtCurrent Go.vi"("axis names"=string[] ["X", "Y"], "Speed"=20.0, "distances"=dbl[] [2.64, 9.09], "Motion in"=w312) -> ("Motion out"=w313:refnum<class "Motion.lvclass">)  [unwired: 6 in, 1 out]
              n112 = Build Array(2.64 ("element"), 9.09 ("element")) -> (w328:dbl[])
              n113 = Concatenate Strings("Bottom right of Chip  " ("string"), w339) -> (w317:string)
              n114 = call "Joystick and Camera SHIH VPC- external Connection.vi"("Motion in"=w313, "Measurement Point"=w317, "Inital GO"=FALSE) -> ("Motion out"=w315:refnum<class "Motion.lvclass">, "Sum"=w314:dbl[])  [unwired: 4 in, 2 out]
              n115 = call "XYtoRPHI.vi"("X-Y"=w328) -> ("r-phi"=w330:dbl[])
              n116 = Subtract(x=w314, y=w338) -> (x-y=w331:dbl[])
              n117 = Add(x=w338, y=w314) -> (x+y=w343:dbl[])
              n118 = Index Array(array=w330, index=1) -> (element=w325:dbl)
              n119 = call "XYtoRPHI.vi"("X-Y"=w331) -> ("r-phi"=w342:dbl[])
              n120 = Divide(x=w343, y=2.0) -> (x/y=w337:dbl[])
              n121 = Index Array(array=w342, index=1) -> (element=w326:dbl)
              n122 = Subtract(x=w326, y=w325) -> (x-y=w327:dbl)
              n123 = Replace Array Subset(array=w337, new element=w327, index=3) -> (w335:dbl[])
            }
          }
        }
        "Array 2" <- w240
      }
      event "Measure Pickup Tools": Value Change {
        (unwired) "Measuring Pickup Tools" ("String")
        n124 = event-data() -> ()  [unwired: 1 in, 6 out]
        n125 = Select(t=i8 1, s=w359, f=w358) -> (s? t:f=w360:i32)
        n126 = for {
          N: w360 -> [_]
          tunnel: [w388] -> w362 mode=indexing
          tunnel: w363 -> [w392]
          tunnel: [w374] -> w361
          tunnel: w357 -> [w373] mode=indexing
          # "Default size and\norientation"
          n127 = call "Joystick and Camera SHIH VPC- external Connection.vi"("Motion in"=w392, "XYZTheta"=w373, "Measurement Point"="PickUp tool TopLeft") -> ("Motion out"=w368:refnum<class "Motion.lvclass">, "Sum"=w391:dbl[])  [unwired: 4 in, 2 out]
          n128 = Build Array(0.0 ("element"), 29.94 ("element"), 0.0 ("element"), 0.0 ("element")) -> (w379:dbl[])
          n129 = Add(x=w391, y=w379) -> (x+y=w365:dbl[])
          n130 = Array Subset(array=w365, index=0, length=2) -> (w366:dbl[])
          n131 = call-dynamic "XY Go.vi"("Speed"=20.0, "XY"=w366, "Motion in"=w368) -> ("Motion out"=w367:refnum<class "Motion.lvclass">)  [unwired: 7 in, 1 out]
          n132 = call "Joystick and Camera SHIH VPC- external Connection.vi"("Motion in"=w367, "Measurement Point"="PickUp tool BottomRight", "Inital GO"=FALSE) -> ("Motion out"=w374:refnum<class "Motion.lvclass">, "Sum"=w390:dbl[])  [unwired: 4 in, 2 out]
          n133 = Add(x=w391, y=w390) -> (x+y=w397:dbl[])
          n134 = Subtract(x=w390, y=w391) -> (x-y=w389:dbl[])
          n135 = Divide(x=w397, y=2.0) -> (x/y=w394:dbl[])
          n136 = call "XYtoRPHI.vi"("X-Y"=w389) -> ("r-phi"=w395:dbl[])
          n137 = Index Array(array=w395, index=1) -> (element=w383:dbl)
          n138 = Absolute Value(x=w383) -> (abs(x)=w386:dbl)
          n139 = Sign(1:w383) -> (0:w384:dbl)
          n140 = Subtract(x=w386, y=1.5707963267948966) -> (x-y=w385:dbl)
          n141 = Multiply(x=w384, y=w385) -> (x*y=w382:dbl)
          n142 = Replace Array Subset(array=w394, new element=w382, index=3) -> (w388:dbl[])
        }
        "Measured PickupTool position" <- w362
      }
      event "Deposit Glue": Value Change {
        # "glue box (half-width, half-length, lines)"
        # "Sensor glue pattern Sensor A then B"
        # "Unmount syringe"
        # "first needle park position\nneedle gap on Z value : 0.5 mm"
        # "Syringe-camera offset"
        n143 = event-data() -> ()  [unwired: 1 in, 6 out]
        n144 = call-poly <vilib>:"Read Delimited Spreadsheet.vi"("file path (dialog if empty)"=path "D:/INTT/V1/Assembly Data/Tool Offsets/Dispense Tip Offset.txt", "number of rows (all:-1)"=-1) -> ("first row"=w451:dbl[])  [unwired: 8 in, 5 out]
        n145 = Build Array(11.75, -22, 0.5 ("element"), 0.0 ("element")) -> (w444:dbl[])
        n146 = Index Array(array=w451, index #1=0 ("index"), index #2=1 ("index")) -> (element #1=w446:dbl, element #2=w443:dbl)
        n147 = Build Array(w446, w443, 0.0 ("element"), 0.0 ("element")) -> (w424:dbl[])
        n148 = Add(x=w424, y=w444) -> (x+y=w411:dbl[])
        n149 = Add(x=w412, y=w411) -> (x+y=w430:dbl[])
        "Needle parking position" <- w430
        n150 = call "XYZTheta Go.vi"("XYZTheta In"=w430, "Motion in"=w431) -> ("error out"=w442:errorcluster, "XYZTheta Out"=w440:dbl[], "Motion out"=w429:refnum<class "Motion.lvclass">)  [unwired: 7 in]
        n151 = call "Display Message to User"("error in (no error)"=w442) -> ("error out"=w432:errorcluster)  [unwired: 9 in, 1 out]
        n152 = Select(t=dbl[][] [[-8.43, -62.0, 4.0, 4.0], [-5.62, -59.0, 4.0, 4.0], [-2.81, -56.0, 4.0, 4.0], [0.0, -53.0, 1.0, 1.0], [-8.43, -48.0, 4.0, 0.0], [-5.62, -45.0, 4.0, 0.0], [-2.81, -42.0, 4.0, 0.0], [0.0, -39.0, 1.0, 0.0]], s=w406, f=dbl[][] [[-8.43, -48.0, 4.0, 4.0], [-5.62, -45.0, 4.0, 4.0], [-2.81, -42.0, 4.0, 4.0], [0.0, -39.0, 1.0, 1.0], [-8.43, -62.0, 4.0, 0.0], [-5.62, -59.0, 4.0, 0.0], [-2.81, -56.0, 4.0, 0.0], [0.0, -53.0, 1.0, 0.0]]) -> (s? t:f=w403:dbl[][])
        n153 = Index Array(array=w440, index=2) -> (element=w436:dbl)
        n154 = call-dynamic "Z Go.vi"("error in (no error)"=w432, "Speed"=20.0, "Position"=0.0, "Motion in"=w429) -> ("error out"=w428:errorcluster, "Motion out"=w435:refnum<class "Motion.lvclass">)  [unwired: 6 in]
        n155 = call "Display Message to User2"("error in (no error)"=w428) -> ("error out"=w427:errorcluster)  [unwired: 9 in, 1 out]
        n156 = Add(x=w436, y=-2.5) -> (x+y=w437:dbl)
        n157 = call-dynamic "Z Go.vi"("error in (no error)"=w427, "Speed"=20.0, "Position"=w437, "Motion in"=w435) -> ("error out"=w425:errorcluster, "Motion out"=w426:refnum<class "Motion.lvclass">)  [unwired: 6 in]
        n158 = call-dynamic "Connect.vi"("Ultimus V in"=refnum<class "Ultimus V2.lvclass"> refnum ("Ultimus V2.lvclass")) -> ("Ultimus V out"=w423:refnum<class "Ultimus V2.lvclass">)  [unwired: 9 in, 1 out]
        n159 = case shown="True" w415 {
          tunnel: w426 -> [w467 w570]
          tunnel: w425 -> [w468 w569]
          tunnel: [w466 w568] -> w420
          tunnel: [w468 w567] -> w418
          tunnel: w414 -> [w463 w561]
          tunnel: w424 -> [w462 w566]
          tunnel: w423 -> [w464 w565]
          tunnel: [w465 w564] -> w421
          tunnel: w413 -> [w461 w563]
          tunnel: w403 -> [w460 _]
          tunnel: "Needle Height Compenstation\n(glue gap)" -> [w459 w562]
          tunnel: "check height?" -> [w458 w559]
          tunnel: "Ultimus Pressure" -> [w457 w558]
          frame False {
            # "two sensor, Sensor B then A"
            n160 = for {
              N: w461 -> [_]
              tunnel: w467 -> [w485]
              tunnel: [w484] -> w465
              tunnel: [w483] -> w466
              tunnel: w464 -> [w482]
              tunnel: w463 -> [w481] mode=indexing
              tunnel: w462 -> [w475]
              tunnel: w460 -> [w477]
              tunnel: w459 -> [w471]
              tunnel: w458 -> [w470]
              tunnel: w457 -> [w469]
              i -> [w473]
              # "four\nloops"
              n161 = Multiply(x=4, y=w473) -> (x*y=w472:i32)
              n162 = Array Subset(array=w477, index (row)=w472, length (row)=4 ("length"), index (col)=0, length (col)=3 ("length")) -> (w476:dbl[][])
              "GlueBox" <- w476
              n163 = for {
                N: 4 -> [_]
                tunnel: w485 -> [w545]
                tunnel: [w537] -> w484
                tunnel: [w532] -> w483
                tunnel: w482 -> [w524]
                tunnel: w481 -> [w502]
                tunnel: w476 -> [w499] mode=indexing
                tunnel: w475 -> [w505]
                tunnel: w471 -> [w491]
                tunnel: w470 -> [w488]
                tunnel: w469 -> [w487]
                n164 = Index Array(array=w499, index=0) -> (element=w521:dbl)
                n165 = Index Array(array=w499, index=1) -> (element=w520:dbl)
                n166 = Array Subset(array=w502, index=0, length=2) -> (w504:dbl[])
                n167 = Add(x=w504, y=w505) -> (x+y=w503:dbl[])
                n168 = Absolute Value(x=w521) -> (abs(x)=w519:dbl)
                n169 = Absolute Value(x=w520) -> (abs(x)=w517:dbl)
                n170 = Add(x=w503, y=w499) -> (x+y=w514:dbl[])
                n171 = Multiply(x=w517, y=2.0) -> (x*y=w495:dbl)
                n172 = Multiply(x=w519, y=2.0) -> (x*y=w496:dbl)
                n173 = Multiply(x=w495, y=-1.0) -> (x*y=w507:dbl)
                n174 = Build Array(0.0 ("element"), w495) -> (w515:dbl[])
                n175 = Build Array(w496, 0.0 ("element")) -> (w512:dbl[])
                n176 = Build Array(0.0 ("element"), w507) -> (w493:dbl[])
                n177 = Add(x=w514, y=w515) -> (x+y=w511:dbl[])
                n178 = Add(x=w511, y=w512) -> (x+y=w494:dbl[])
                n179 = call-dynamic "XY Go.vi"("Speed"=200.0, "XY"=w514, "Motion in"=w545) -> ("error out"=w497:errorcluster, "Motion out"=w544:refnum<class "Motion.lvclass">)  [unwired: 7 in]
                n180 = Add(x=w494, y=w493) -> (x+y=w492:dbl[])
                n181 = Index Array(array=w502, index=2) -> (element=w501:dbl)
                n182 = Index Array(array=w499, index=2) -> (element=w498:dbl)
                n183 = Add(x=w501, y=w491) -> (x+y=w530:dbl)
                n184 = Build Array(w511, w494, w492, w514) -> (w506:dbl[][])
                "appended array" <- w506
                n185 = call-dynamic "Z Go.vi"("error in (no error)"=w497, "Speed"=5.0, "Position"=w530, "Motion in"=w544) -> ("error out"=w490:errorcluster, "Motion out"=w540:refnum<class "Motion.lvclass">)  [unwired: 6 in]
                n186 = case shown="True" w488 {
                  tunnel: w490 -> [w549 w551]
                  tunnel: [w549 w550] -> w489
                  frame False {
                  }
                  frame True {
                    n187 = call "Display Message to User11"("error in (no error)"=w551) -> ("error out"=w550:errorcluster)  [unwired: 9 in, 1 out]
                  }
                }
                n188 = call "vacuum.vi"("error in (no error)"=w489, "Vacuum Setting (0000)"=i64 100, "Ultimus V in"=w524) -> ("error out"=w542:errorcluster, "Ultimus V out"=w527:refnum<class "Ultimus V2.lvclass">)  [unwired: 7 in]
                n189 = call-dynamic "Pressure.vi"("error in (no error)"=w542, "Pressure"=w487, "Ultimus V in"=w527) -> ("error out"=w543:errorcluster, "Ultimus V out"=w526:refnum<class "Ultimus V2.lvclass">)  [unwired: 7 in]
                n190 = call-dynamic "Dispense.vi"("error in (no error)"=w543, "Ultimus V in"=w526) -> ("error out"=w539:errorcluster, "Ultimus V out"=w525:refnum<class "Ultimus V2.lvclass">)  [unwired: 8 in]
                n191 = for {
                  N: w498 -> [_]
                  tunnel: w540 -> [w557]
                  tunnel: w539 -> [w556]
                  tunnel: [w555] -> w538
                  tunnel: [w554] -> w536
                  tunnel: w506 -> [w553] mode=indexing
                  (unwired) 4.5 ("Speed")
                  n192 = call-dynamic "XY Go.vi"("error in (no error)"=w556, "Speed"=4.5, "XY"=w553, "Motion in"=w557) -> ("error out"=w555:errorcluster, "Motion out"=w554:refnum<class "Motion.lvclass">)  [unwired: 6 in]
                }
                n193 = Add(x=w530, y=-2.0) -> (x+y=w533:dbl)
                n194 = call-dynamic "Dispense.vi"("error in (no error)"=w538, "Ultimus V in"=w525) -> ("error out"=w531:errorcluster, "Ultimus V out"=w537:refnum<class "Ultimus V2.lvclass">)  [unwired: 8 in]
                n195 = call-dynamic "Z Go.vi"("error in (no error)"=w531, "Speed"=10.0, "Position"=w533, "Motion in"=w536) -> ("Motion out"=w532:refnum<class "Motion.lvclass">)  [unwired: 6 in, 1 out]
              }
            }
          }
          frame True {
            n196 = case shown="True" w559 {
              tunnel: w561 -> [w571 w575]
              tunnel: [w571 w572] -> w560
              frame False {
              }
              frame True {
                n197 = Array Subset(array=w575, index (row)=12 ("index"), length (row)=4 ("length")) -> (w572:dbl[][])  [unwired: 2 in]
              }
            }
            n198 = for {
              N: w563 -> [_]
              tunnel: w570 -> [w619]
              tunnel: w569 -> [w618]
              tunnel: [w608] -> w564
              tunnel: [w607] -> w568
              tunnel: [w606] -> w567
              tunnel: w560 -> [w594] mode=indexing
              tunnel: w566 -> [w593]
              tunnel: w565 -> [w592]
              tunnel: w562 -> [w590]
              tunnel: w559 -> [w587]
              tunnel: w558 -> [_]
              shift-right: [w581] -> _
              shift-left: _ -> [w580]
              i -> [w578]
              # "move the glue in x-dir\n0.1 mm closer to center"
              n199 = Quotient & Remainder(x=w578, y="glue deposit group") -> (x-y*floor(x/y)=w579:i32)  [unwired: 1 out]
              n200 = Equal To 0?(x=w579) -> (x = 0?=w586:bool)
              n201 = Index Array(array=w594, index=2) -> (element=w595:dbl)
              n202 = Add(x=w594, y=w593) -> (x+y=w617:dbl[])
              n203 = Build Array(0.0 ("element"), 3.3 ("element")) -> (w622:dbl[])
              n204 = Subtract(x=w617, y=w622) -> (x-y=w623:dbl[])
              n205 = Add(x=w595, y=w590) -> (x+y=w596:dbl)
              n206 = Add(x=w617, y=w622) -> (x+y=w604:dbl[])
              n207 = call-dynamic "XY Go.vi"("error in (no error)"=w618, "Speed"=200.0, "XY"=w623, "Motion in"=w619) -> ("error out"=w609:errorcluster, "Motion out"=w602:refnum<class "Motion.lvclass">)  [unwired: 6 in]
              n208 = call-dynamic "Z Go.vi"("error in (no error)"=w609, "Speed"=5.0, "Position"=w596, "Motion in"=w602) -> ("error out"=w589:errorcluster)  [unwired: 6 in, 1 out]
              n209 = case shown="True" w587 {
                tunnel: w589 -> [w646 w648]
                tunnel: [w646 w647] -> w588
                frame False {
                }
                frame True {
                  n210 = call "Display Message to User7"("error in (no error)"=w648) -> ("error out"=w647:errorcluster)  [unwired: 9 in, 1 out]
                }
              }
              n211 = call "vacuum.vi"("error in (no error)"=w588, "Vacuum Setting (0000)"=i64 100, "Ultimus V in"=w592) -> ("error out"=w582:errorcluster, "Ultimus V out"=w583:refnum<class "Ultimus V2.lvclass">)  [unwired: 7 in]
              n212 = case shown="True" w586 {
                tunnel: [w625 w637] -> w585
                tunnel: [w626 w636] -> w584
                tunnel: w583 -> [w628 w635]
                tunnel: w582 -> [w627 w633]
                tunnel: [w624 w630] -> w581
                tunnel: w580 -> [w624 _]
                tunnel: [w624 w629] -> w576
                frame False {
                  n213 = call-dynamic "Pressure.vi"("error in (no error)"=w627, "Pressure"=w624, "Ultimus V in"=w628) -> ("error out"=w625:errorcluster, "Ultimus V out"=w626:refnum<class "Ultimus V2.lvclass">)  [unwired: 7 in]
                }
                frame True {
                  n214 = flat-sequence {
                    tunnel: [w640] -> _
                    tunnel: w635 -> [w640]
                    tunnel: [w640] -> w634
                    tunnel: w633 -> [w639]
                    tunnel: [w639] -> w632
                    tunnel: [w638] -> w631
                    tunnel: [w638] -> w630
                    tunnel: [w645] -> w637
                    tunnel: [w644] -> w636
                    tunnel: w634 -> [w643]
                    tunnel: w632 -> [w642]
                    tunnel: w631 -> [w641]
                    tunnel: [w641] -> w629
                    frame #0 {
                      n215 = call "air pressure setting.vi"() -> ("air pressure indecator"=w638:i32)  [unwired: 1 out]
                    }
                    frame #1 {
                      n216 = call-dynamic "Pressure.vi"("error in (no error)"=w642, "Pressure"=w641, "Ultimus V in"=w643) -> ("error out"=w645:errorcluster, "Ultimus V out"=w644:refnum<class "Ultimus V2.lvclass">)  [unwired: 7 in]
                    }
                  }
                }
              }
              "air pressure indecator" <- w576
              n217 = call-dynamic "Dispense.vi"("error in (no error)"=w585, "Ultimus V in"=w584) -> ("error out"=w603:errorcluster, "Ultimus V out"=w610:refnum<class "Ultimus V2.lvclass">)  [unwired: 8 in]
              n218 = call "Time Delay"("error in (no error)"=w603) -> ("error out"=w601:errorcluster)  [unwired: 10 in]
              n219 = call-dynamic "XY Go.vi"("error in (no error)"=w601, "Speed"=5.0, "XY"=w604, "Motion in"=w602) -> ("error out"=w600:errorcluster, "Motion out"=w598:refnum<class "Motion.lvclass">)  [unwired: 6 in]
              n220 = call "Time Delay3"("error in (no error)"=w600) -> ("error out"=w599:errorcluster)  [unwired: 10 in]
              n221 = call "Time Delay2"("error in (no error)"=w601) -> ("error out"=w611:errorcluster)  [unwired: 10 in]
              n222 = call-dynamic "Dispense.vi"("error in (no error)"=w611, "Ultimus V in"=w610) -> ("Ultimus V out"=w608:refnum<class "Ultimus V2.lvclass">)  [unwired: 8 in, 1 out]
              n223 = Add(x=w596, y=-2.5) -> (x+y=w614:dbl)
              n224 = call-dynamic "Z Go.vi"("error in (no error)"=w599, "Speed"=10.0, "Position"=w614, "Motion in"=w598) -> ("error out"=w606:errorcluster, "Motion out"=w607:refnum<class "Motion.lvclass">)  [unwired: 6 in]
            }
          }
        }
        n225 = call-dynamic "Disconnect.vi"("Ultimus V in"=w421) -> ()  [unwired: 9 in, 1 out]
        n226 = call "XYZTheta Go.vi"("error in (no error)"=w418, "XYZTheta In"=dbl[] [400.0, 600.0, 0.0, 0.1], "Motion in"=w420) -> ("error out"=w419:errorcluster, "Motion out"=w416:refnum<class "Motion.lvclass">)  [unwired: 6 in, 1 out]
        n227 = call "Display Message to User3"("error in (no error)"=w419) -> ()  [unwired: 9 in, 2 out]
      }
      event "Needle Alignment": Value Change {
        (unwired) "Needle Alignment in progress ...." ("String")
        # "first needle park position\nneedle gap on Z value : 0.5 mm"
        # "Syringe-camera offset"
        n228 = event-data() -> ()  [unwired: 1 in, 6 out]
        n229 = call-poly <vilib>:"Read Delimited Spreadsheet.vi"("file path (dialog if empty)"=path "D:/INTT/V1/Assembly Data/Tool Offsets/Dispense Tip Offset.txt", "number of rows (all:-1)"=-1) -> ("first row"=w689:dbl[])  [unwired: 8 in, 5 out]
        n230 = Build Array(11.75, -22, 0.5 ("element"), 0.0 ("element")) -> (w682:dbl[])
        n231 = Index Array(array=w689, index #1=0 ("index"), index #2=1 ("index")) -> (element #1=w684:dbl, element #2=w681:dbl)
        n232 = Build Array(w684, w681, 0.0 ("element"), 0.0 ("element")) -> (w651:dbl[])
        n233 = Add(x=w651, y=w682) -> (x+y=w675:dbl[])
        n234 = Add(x=w674, y=w675) -> (x+y=w676:dbl[])
        n235 = call "XYZTheta Go.vi"("XYZTheta In"=w676, "Motion in"=w666) -> ("error out"=w680:errorcluster, "XYZTheta Out"=w656:dbl[], "Motion out"=w665:refnum<class "Motion.lvclass">)  [unwired: 7 in]
        n236 = call "Display Message to User10"("error in (no error)"=w680) -> ("error out"=w677:errorcluster)  [unwired: 9 in, 1 out]
        n237 = call-dynamic "Z Go.vi"("error in (no error)"=w677, "Speed"=20.0, "Position"=0.0, "Motion in"=w665) -> ("Motion out"=w664:refnum<class "Motion.lvclass">)  [unwired: 6 in, 1 out]
        n238 = Replace Array Subset(array=w656, new element=0.0 ("new element/subarray"), index=2) -> (w653:dbl[])
        n239 = call "Joystick and Camera SHIH VPC- external Connection.vi"("Motion in"=w664, "XYZTheta"=w653, "Measurement Point"="Touch Needle on a surface") -> ("Motion out"=w662:refnum<class "Motion.lvclass">, "Gantry"=w652:dbl[])  [unwired: 4 in, 2 out]
        n240 = Subtract(x=w652, y=w651) -> (x-y=w650:dbl[])
        n241 = call "Joystick and Camera SHIH VPC- external Connection.vi"("Motion in"=w662, "XYZTheta"=w650, "Measurement Point"="Measure the touch spot with camera") -> ("Motion out"=w658:refnum<class "Motion.lvclass">, "Gantry"=w661:dbl[])  [unwired: 4 in, 2 out]
        n242 = Subtract(x=w652, y=w661) -> (x-y=w660:dbl[])
        n243 = call-poly <vilib>:"Write Delimited Spreadsheet.vi"("file path (dialog if empty)"=path "D:/INTT/V1/Assembly Data/Tool Offsets/Dispense Tip Offset.txt", "1D data"=w660, "append to file? (new file:F)"=FALSE) -> ()  [unwired: 11 in, 2 out]
      }
      event "Pick and place": Value Change {
        (unwired) "PICK and PLACE samples ..." ("String")
        (unwired) -21.3804 ("new element/subarray")
        n244 = event-data() -> ()  [unwired: 1 in, 6 out]
        n245 = call-poly <vilib>:"Read Delimited Spreadsheet.vi"("file path (dialog if empty)"=path "D:/INTT/V1/Assembly Data/Tool Offsets/Bellows Tool Offset.txt", "number of rows (all:-1)"=-1) -> ("first row"=w715:dbl[])  [unwired: 8 in, 5 out]
        n246 = Select(t=1, s=w696, f=w704) -> (s? t:f=w720:i32)
        n247 = Index Array(array=w715, index #1=0 ("index"), index #2=1 ("index"), index #3=2 ("index")) -> (element #1=w711:dbl, element #2=w710:dbl, element #3=w709:dbl)
        n248 = for {
          N: w720 -> [_]
          tunnel: w704 -> [w756]
          tunnel: w705 -> [w752]
          tunnel: w718 -> [w776]
          tunnel: [w764] -> w708
          tunnel: w706 -> [w774] mode=indexing
          tunnel: [w740] -> w700
          tunnel: w699 -> [w727]
          tunnel: w711 -> [w766]
          tunnel: w710 -> [w765]
          tunnel: w707 -> [w749]
          tunnel: w709 -> [w763]
          tunnel: w696 -> [w733]
          tunnel: "VacChannel for sample" -> [w735]
          tunnel: "check height? 2" -> [w728]
          tunnel: w696 -> [w721]
          i -> [w742]
          w725 = 0 ("Channel")
          w724 = TRUE ("Value")
          # "put back pickup tool"
          # "if chips, do one pickup tool and multiple samples;\nif sensors, one pickup tool for one sample ( so 2->2);"
          # "build a fake 2d arrays"
          # "sensor"
          # "chip pickup tool"
          # "pickup tool height offset"
          # "Pick up PICKUP TOOL"
          # "Pick up CHIPs/Sensor and place on HDI"
          n249 = Select(t=w756, s=w733, f=1) -> (s? t:f=w755:i32)
          n250 = Build Array(w766, w765, w763, 0.0 ("element")) -> (w761:dbl[])
          n251 = Add(x=w774, y=w761) -> (x+y=w762:dbl[])
          n252 = call "XYZTheta-2Zspeed Go.vi"("XYZTheta In"=w762, "Motion in"=w776) -> ("error out"=w723:errorcluster, "Motion out"=w775:refnum<class "Motion.lvclass">)  [unwired: 7 in, 1 out]
          n253 = Select(t=-18.52 ("new element/subarray"), s=w733, f=-13.13 ("t")) -> (s? t:f=w757:dbl)
          n254 = call "WriteReadWait.vi"("Read Value"=w724, "Write Value"=w724, "error in (no error)"=w723, "Read"=w725, "Write"=w725, "I-O in"=w727) -> ("error out"=w722:errorcluster, "I-O out"=w726:refnum<class "NI-DAQ.lvclass">)  [unwired: 4 in]
          n255 = Replace Array Subset(array=w761, new element=w757, index=2) -> (w759:dbl[])
          n256 = Index Array(array=w752, index (row)=w742) -> (element=w751:dbl[])  [unwired: 1 in]
          n257 = call "Time Delay8"("error in (no error)"=w722) -> ("error out"=w772:errorcluster)  [unwired: 10 in]
          n258 = Build Array(w751, w751) -> (w750:dbl[][])
          n259 = Select(t=w752, s=w733, f=w750) -> (s? t:f=w753:dbl[][])
          n260 = Index Array(array=w749, index (row)=w742) -> (element=w748:dbl[])  [unwired: 1 in]
          n261 = Build Array(w748, w748) -> (w747:dbl[][])
          n262 = Select(t=w749, s=w733, f=w747) -> (s? t:f=w730:dbl[][])
          n263 = case shown="True" w728 {
            tunnel: [w777 w779] -> w729
            tunnel: w730 -> [w777 w778]
            frame False {
            }
            frame True {
              n264 = Array Subset(array=w778, index (row)=12 ("index"), length (row)=4 ("length")) -> (w779:dbl[][])  [unwired: 2 in]
            }
          }
          n265 = Select(t="chip placement height compensation", s=w733, f=0.0) -> (s? t:f=w731:dbl)
          n266 = for {
            N: w755 -> [_]
            tunnel: w753 -> [w795] mode=indexing
            tunnel: w775 -> [w797]
            tunnel: w759 -> [w796]
            tunnel: w772 -> [w794]
            tunnel: [w793] -> w767
            tunnel: w726 -> [w792]
            tunnel: w729 -> [w789] mode=indexing
            tunnel: [w788] -> w758
            tunnel: w731 -> [w787]
            tunnel: w735 -> [w786]
            tunnel: [w785] -> w734
            tunnel: w733 -> [w784]
            tunnel: w728 -> [w783]
            tunnel: w721 -> [w782]
            n267 = flat-sequence {
              tunnel: w795 -> [w810]
              tunnel: [w812] -> w798
              tunnel: w797 -> [w811]
              tunnel: w796 -> [w809]
              tunnel: w794 -> [w807]
              tunnel: w792 -> [w800]
              tunnel: [w804] -> w791
              tunnel: [w805] -> w790
              tunnel: w786 -> [w802]
              tunnel: w798 -> [w839]
              tunnel: [w838] -> w793
              tunnel: w796 -> [w836]
              tunnel: w791 -> [w837]
              tunnel: w790 -> [w825]
              tunnel: w789 -> [w835]
              tunnel: [w819] -> w788
              tunnel: w787 -> [w829]
              tunnel: w786 -> [w824]
              tunnel: [w820] -> w785
              tunnel: w784 -> [_]
              tunnel: w783 -> [w826]
              tunnel: w782 -> [w818]
              frame #0 {
                w803 = TRUE ("Value")
                # "pickup sample"
                # "pickup sample from tray"
                n268 = Add(x=w810, y=w809) -> (x+y=w808:dbl[])
                n269 = call "XYZTheta-2Zspeed Go.vi"("error in (no error)"=w807, "XYZTheta In"=w808, "Motion in"=w811) -> ("error out"=w806:errorcluster, "Motion out"=w812:refnum<class "Motion.lvclass">)  [unwired: 6 in, 1 out]
                n270 = call "Time Delay4"("error in (no error)"=w806) -> ("error out"=w799:errorcluster)  [unwired: 10 in]
                n271 = call "Time Delay11"("error in (no error)"=w799) -> ("error out"=w801:errorcluster)  [unwired: 10 in]
                n272 = call "WriteReadWait.vi"("Read Value"=w803, "Write Value"=w803, "error in (no error)"=w801, "Read"=w802, "Write"=w802, "I-O in"=w800) -> ("error out"=w804:errorcluster, "I-O out"=w805:refnum<class "NI-DAQ.lvclass">)  [unwired: 4 in]
              }
              frame #1 {
                w822 = FALSE ("Value")
                # "place chip on HDI"
                # "release sample on HDI"
                # "lift for chip/sensor thickness"
                # "place sample on HDI"
                n273 = Add(x=w835, y=w836) -> (x+y=w831:dbl[])
                n274 = Build Array(0.0 ("element"), 0.0 ("element"), w829, 0.0 ("element")) -> (w830:dbl[])
                n275 = Add(x=w831, y=w830) -> (x+y=w815:dbl[])
                n276 = call-poly <vilib>:"Read Delimited Spreadsheet.vi"("file path (dialog if empty)"=path "D:/INTT/V1/Assembly Data/Tool Offsets/chip_place_Zoffset.txt", "number of rows (all:-1)"=-1) -> ("first row"=w814:dbl[])  [unwired: 8 in, 5 out]
                "chip place Z offset" <- w814
                n277 = Add(x=w814, y=w815) -> (x+y=w813:dbl[])
                n278 = call "XYZTheta-2Zspeed Go.vi"("error in (no error)"=w837, "XYZTheta In"=w813, "Motion in"=w839) -> ("error out"=w828:errorcluster, "Motion out"=w838:refnum<class "Motion.lvclass">)  [unwired: 6 in, 1 out]
                n279 = case shown="True" w826 {
                  tunnel: w828 -> [w844 w846]
                  tunnel: [w844 w845] -> w827
                  frame False {
                  }
                  frame True {
                    n280 = call "Display Message to User6"("error in (no error)"=w846) -> ("error out"=w845:errorcluster)  [unwired: 9 in, 1 out]
                  }
                }
                n281 = case shown="True" w818 {
                  tunnel: w827 -> [w841 w843]
                  tunnel: [w840 w842] -> w823
                  frame False {
                    n282 = call "Time Delay7"("error in (no error)"=w841) -> ("error out"=w840:errorcluster)  [unwired: 10 in]
                  }
                  frame True {
                    n283 = call "Time Delay6"("error in (no error)"=w843) -> ("error out"=w842:errorcluster)  [unwired: 10 in]
                  }
                }
                n284 = call "WriteReadWait.vi"("Read Value"=w822, "Write Value"=w822, "error in (no error)"=w823, "Read"=w824, "Write"=w824, "I-O in"=w825) -> ("error out"=w821:errorcluster, "I-O out"=w820:refnum<class "NI-DAQ.lvclass">)  [unwired: 4 in]
                n285 = call "Time Delay5"("error in (no error)"=w821) -> ("error out"=w819:errorcluster)  [unwired: 10 in]
              }
            }
          }
          n286 = call "XYZTheta-2Zspeed Go.vi"("error in (no error)"=w758, "XYZTheta In"=w762, "Motion in"=w767) -> ("error out"=w732:errorcluster, "Motion out"=w771:refnum<class "Motion.lvclass">)  [unwired: 6 in, 1 out]
          n287 = call "Time Delay9"("error in (no error)"=w732) -> ("error out"=w738:errorcluster)  [unwired: 10 in]
          n288 = call-dynamic "Digital Write 1 Channel.vi"("DAQ Module"=0, "error constant"=w738, "Value"=FALSE, "Channel"=0, "NI-DAQ.lvclass"=w734) -> ("error IO"=w741:errorcluster, "NI-DAQ.lvclass 2"=w740:refnum<class "NI-DAQ.lvclass">)  [unwired: 5 in]
          n289 = call "Time Delay10"("error in (no error)"=w741) -> ("error out"=w768:errorcluster)  [unwired: 10 in]
          n290 = call-dynamic "Z Go.vi"("error in (no error)"=w768, "Speed"=20.0, "Position"=0.0 ("new element/subarray"), "Motion in"=w771) -> ("Motion out"=w764:refnum<class "Motion.lvclass">)  [unwired: 6 in, 1 out]
        }
      }
      event "GOTO": Value Change {
        (unwired) "GOING to a position" ("String")
        n291 = event-data() -> ()  [unwired: 1 in, 6 out]
        n292 = call "XYZTheta-2Zspeed Go.vi"("XYZTheta In"="Parking position", "Motion in"=w849) -> ("Motion out"=w848:refnum<class "Motion.lvclass">)  [unwired: 7 in, 2 out]
      }
      event "READ Position": Value Change {
        n293 = event-data() -> ()  [unwired: 1 in, 6 out]
        n294 = call-dynamic "Get Current Position.vi"("Motion in"=w870) -> ("XYZTheta Out"=→"Gantry current position":dbl[], "Motion out"=w869:refnum<class "Motion.lvclass">)  [unwired: 8 in, 1 out]
      }
      event Timeout {
        n295 = event-data() -> ()  [unwired: 1 in, 3 out]
      }
    }
    "Measure HDI top-left" <- w33
    "Sample on HDI" <- w11
    n296 = feedback-in #1(w31) -> ()
    n297 = feedback-in #2(w33) -> ()
    n298 = feedback-in #3(w28) -> ()
    n299 = feedback-in #4(w20) -> ()
    n300 = feedback-in #5(w17) -> ()
    n301 = feedback-in #6(w25) -> ()
    n302 = feedback-in #7(w11) -> ()
    n303 = feedback-in #8(w26) -> ()
    "# of tasks excuted" <- w22
  }
  n304 = call-dynamic "Disconnect.vi"("I-O in"=w1) -> ()  [unwired: 9 in, 1 out]
  n305 = call-dynamic "Disconnect.vi"("Controller in"=w4) -> ()  [unwired: 9 in, 1 out]
